vi "transfer char run_subvi_14_2014 05 29_JWa.vi"(0 "VISA session":refnum<visa-resource-name>="GPIB0::17::INSTR", 1 "Y2 axis settings":T5={"Y2 axis on/off"=FALSE, "MINIMUM"=0.0, "MAXIMUM"=1.0, "Variable name"="Ig", "LIN or LOG axis"="LIN"} {"MAXIMUM" format="%.9f"; "MINIMUM" format="%.9f"}, 3 "LKG Path":path, 5 "Var1 sweep settings":T7={"start"=40.0, "stop"=-40.0, "step (linear only)"=-1.0, "sweep spacing (linear: 0)"=0, "sweep mode"=FALSE, "compliance (V)"=100.0, "compliance (A)"=0.001} {"compliance (A)" format="%^.2e"; "compliance (V)" format="%.2f"; "sweep spacing (linear: 0)" items=["linear", "log 10", "log 25", "log 50"]; "step (linear only)" format="%.2f"; "stop" format="%.2f"; "start" format="%.2f"}, 7 "Var2 step settings":T6={"compliance (A)"=0.001, "compliance (V)"=100.0, "start"=-2.0, "total points"=2, "step"=-38.0} {"step" format="%.2f"; "start" format="%.2f"; "compliance (V)" format="%.2f"; "compliance (A)" format="%^.2e"}, 9 "integration time":u32(slide) scale=0.0..2.0, 11 "Input Path":path, 12 "Dielectric Constant":dbl=5.0, 13 "Sample Properties:":T4 {"Date Created" format="%<%x>T"}) -> (2 "Check Cluster":T2, 4 "Output":T3 {"Mobility-Lin" format="%#_4e"; "Mobility-Sat" format="%#_4e"}, 6 "Graph Cluster":T1, 15 "error?":errorcluster)   [LabVIEW 2012]
uses:
  <vilib>/Utility/file.llb/Write To Spreadsheet File (DBL).vi
panel:
  out "concatenated string":string
  in  "Output Path":path
  in  "Temp (K)":dbl=0.001 format="%^.2e"
  in  "NumPts":dbl=5.0
  out "Numeric":dbl
  out "min r":dbl
  out "max r":dbl
  out "error? 2":errorcluster
  in  "MAXIMUM":ext format="%.2e"
  in  "MINIMUM":ext=-1e-05 format="%_2e"
  out "Gate Current Plot":cluster{"trace":dbl[], "trace":dbl[]}(graph)
  in  "Y1 axis":string="Id"
  out "graphic display":cluster{"trace":dbl[], "trace":dbl[]}(graph)
  in  "wait time parameter":dbl=1.0
  in  "Value (Either V or A) 4":dbl
  in  "Value (Either V or A) 3":dbl
  in  "Value (Either V or A) 2":dbl
  in  "Value (V or A)":dbl
  in  "compliance (A)":dbl=0.001 format="%^.2e"
  in  "compliance (V)":dbl=100.0 format="%^.2e"
  in  "Iname":string="Is"
  in  "Vname":string="Vs"
  in  "Function":u16(ring)=4 items=["disabled", "Var1", "Var2", "Var1'", "Constant"]
  in  "Mode":u16(ring)=4 items=["V", "I", "VPulse", "IPulse", "Common"]
  in  "Iname 4":string="I4"
  in  "Vname 4":string="V4"
  in  "Function 4":u16(ring)=4 items=["disabled", "Var1", "Var2", "Var1'", "Constant"]
  in  "Mode 4":u16(ring) items=["V", "I", "VPulse", "IPulse", "Common"]
  in  "Iname 3":string="Ig"
  in  "Vname 3":string="Vg"
  in  "Function 3":u16(ring)=1 items=["disabled", "Var1", "Var2", "Var1'", "Constant"]
  in  "Mode 3":u16(ring) items=["V", "I", "VPulse", "IPulse", "Common"]
  in  "Iname 2":string="Id"
  in  "Vname 2":string="Vd"
  in  "Function 2":u16(ring)=2 items=["disabled", "Var1", "Var2", "Var1'", "Constant"]
  in  "Mode 2":u16(ring) items=["V", "I", "VPulse", "IPulse", "Common"]
  in  "reset":bool=TRUE
  # "SMU1"
  # "SMU2"
  # "SMU3"
  # "SMU4"
  # "Sample Properties:"
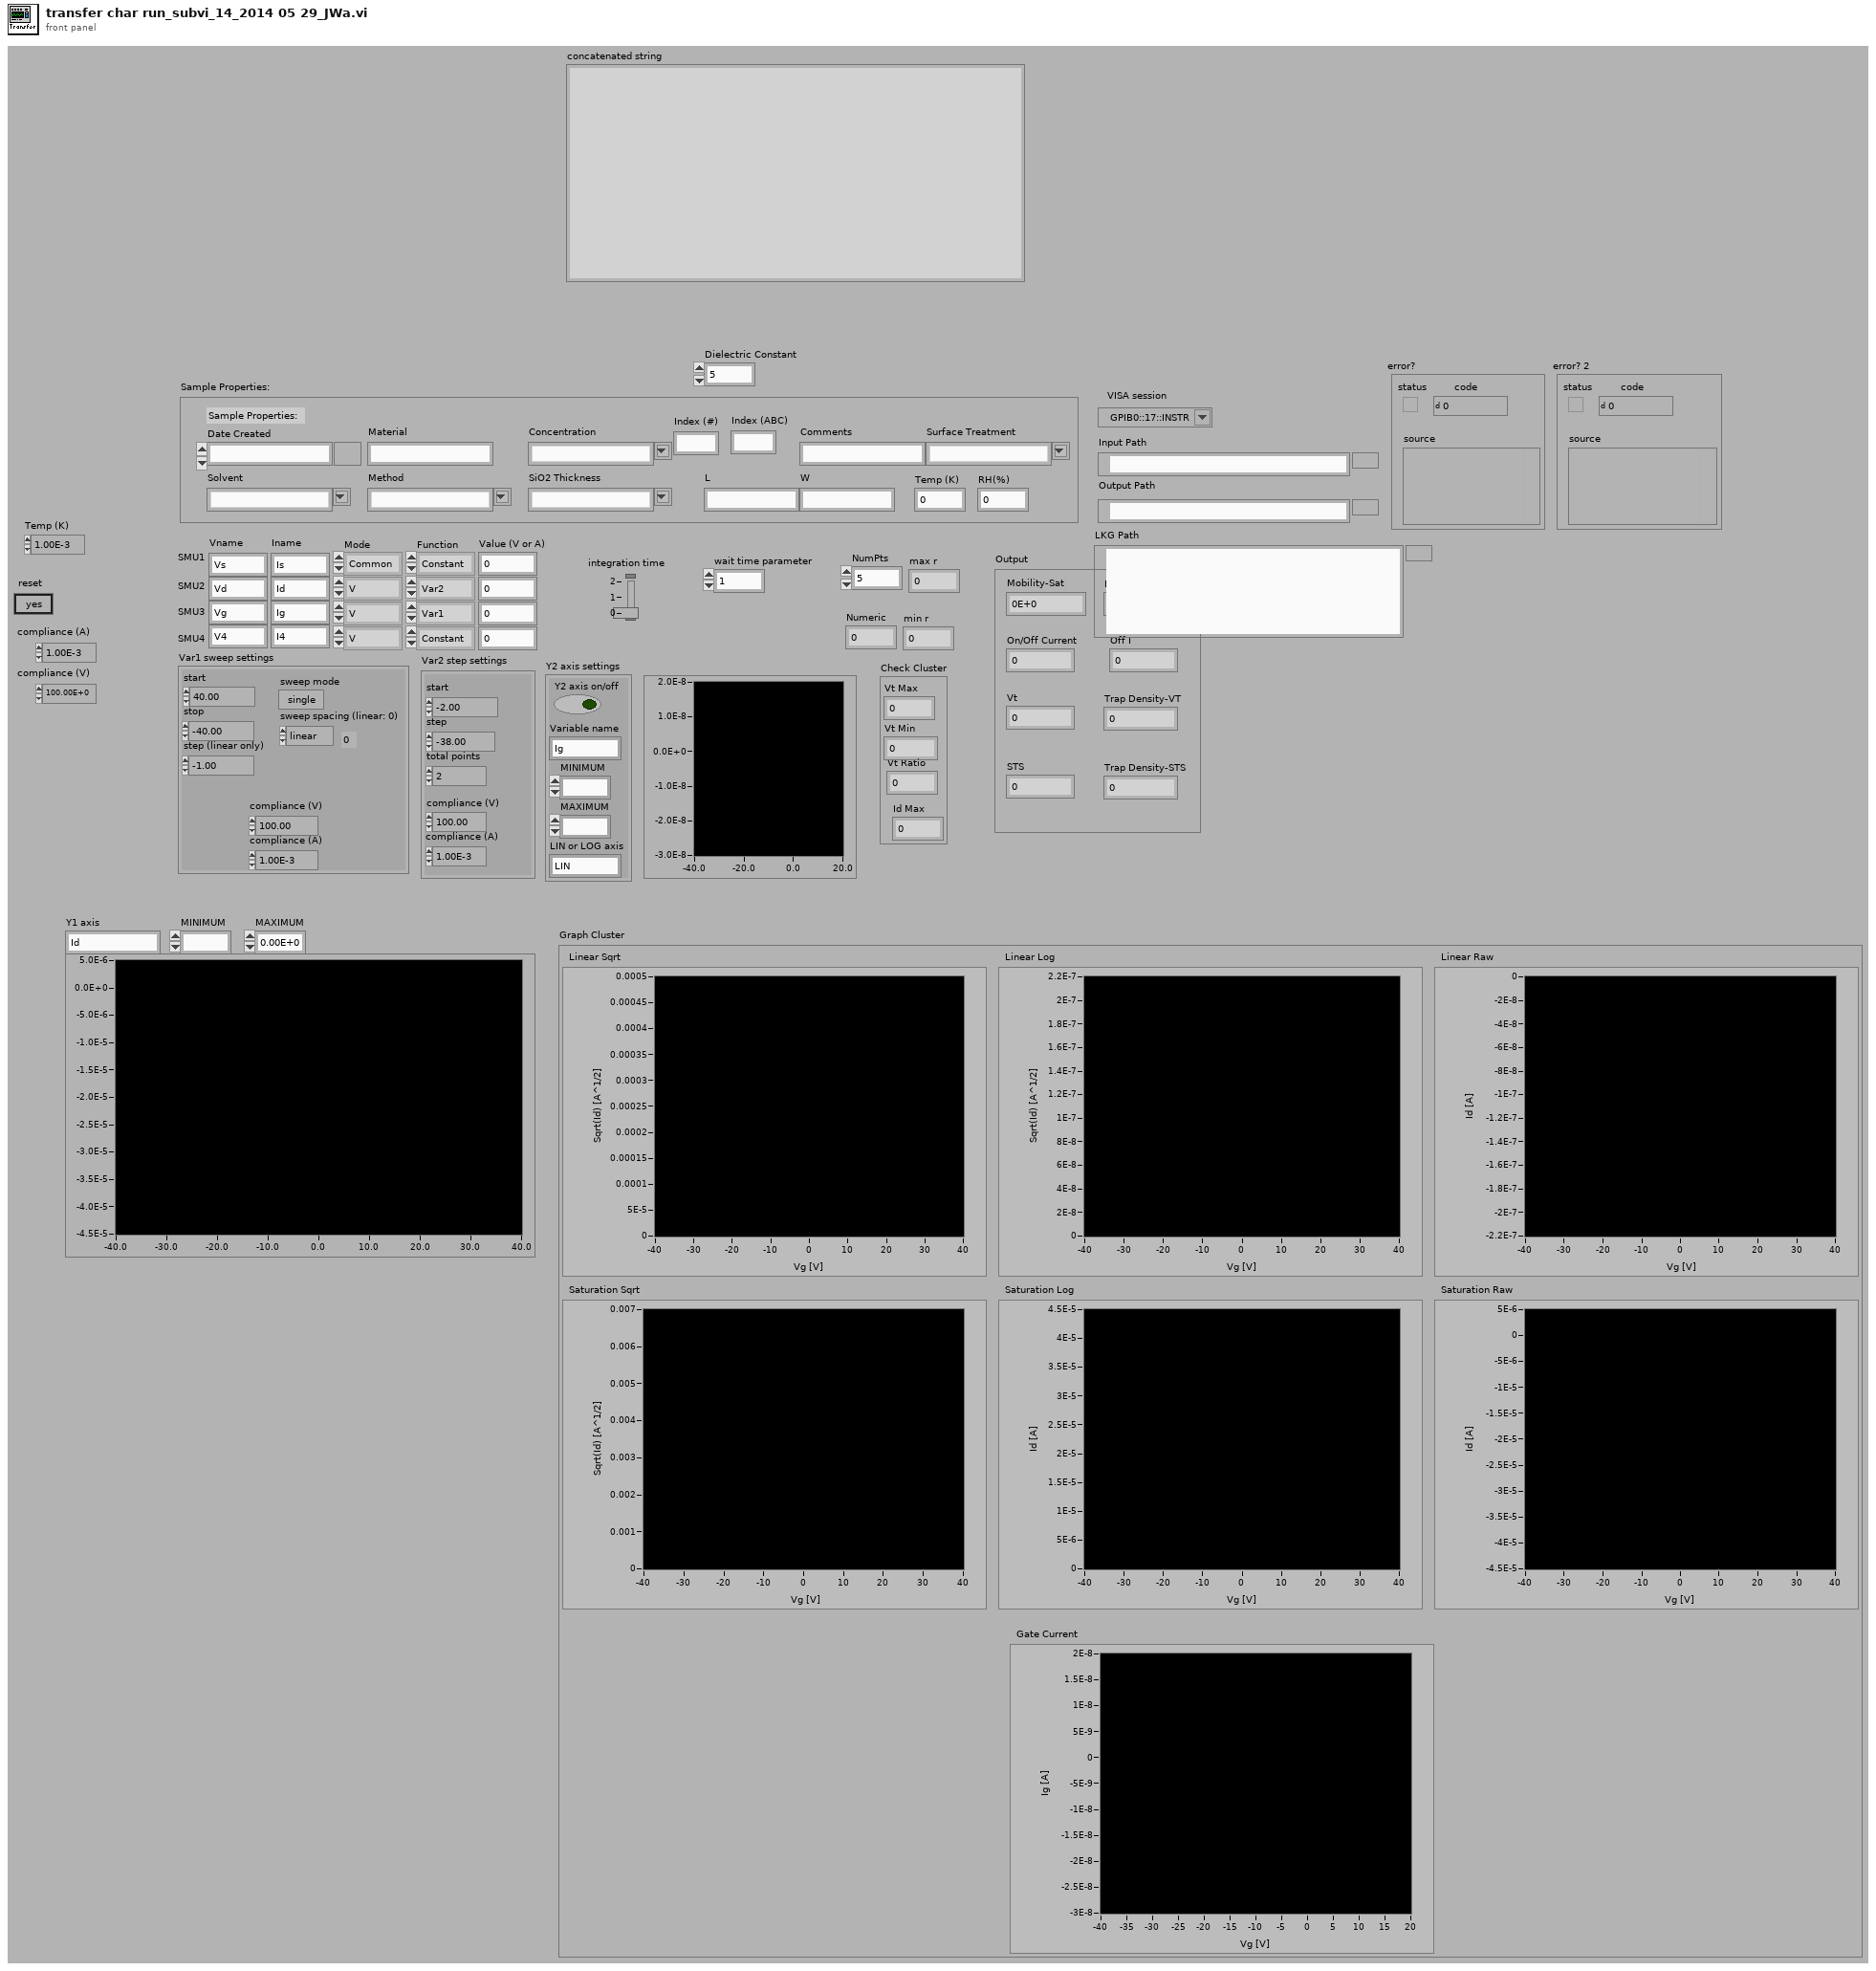
[diagram p1: front panel]
types:
  T1 = cluster{"Linear Sqrt":cluster{dbl[], "trace":dbl[]}[], "Linear Log":cluster{dbl[], "trace":dbl[]}[], "Linear Raw":cluster{dbl[], dbl[]}[], "Saturation Sqrt":cluster{dbl[], "trace":dbl[]}[], "Saturation Log":cluster{dbl[], "trace":dbl[]}[], "Saturation Raw":cluster{dbl[], "trace":dbl[]}[], "Gate Current":cluster{dbl[], "trace":dbl[]}[]}
  T2 = cluster{"Vt Max":i32, "Vt Min":i32, "Vt Ratio":i32, "Id Max":dbl}
  T3 = cluster{"Mobility-Sat":dbl, "Mobility-Lin":dbl, "On/Off Current":dbl, "Off I":dbl, "Vt":dbl, "STS":dbl, "Trap Density-VT":dbl, "Trap Density-STS":dbl}
  T4 = cluster{"Date Created":timestamp, "Material":string, "Solvent":string, "Concentration":string, "Method":string, "SiO2 Thickness":string, "Index (#)":string, "Index (ABC)":string, "L":string, "W":string, "Surface Treatment":string, "Comments":string, "Temp (K)":dbl, "RH(%)":dbl}
  T5 = cluster{"Y2 axis on/off":bool, "MINIMUM":ext, "MAXIMUM":ext, "Variable name":string, "LIN or LOG axis":string}
  T6 = cluster{"compliance (A)":dbl, "compliance (V)":dbl, "start":dbl, "total points":u16, "step":dbl}
  T7 = cluster{"start":dbl, "stop":dbl, "step (linear only)":dbl, "sweep spacing (linear: 0)":u16, "sweep mode":bool, "compliance (V)":dbl, "compliance (A)":dbl}
  T8 = cluster{"Vt Max":dbl, "Vt Min":dbl, "Vt Ratio":dbl, "Id Max":dbl}
  T9 = cluster{"Mobility-Sat":dbl, "Mobility-Lin":dbl, "On/Off I-Sat":dbl, "Off I-Sat":dbl, "VT-Sat":dbl, "Sub Threshold Swing":dbl, "Trap Density-VT":dbl, "Trap Density (N)":dbl}
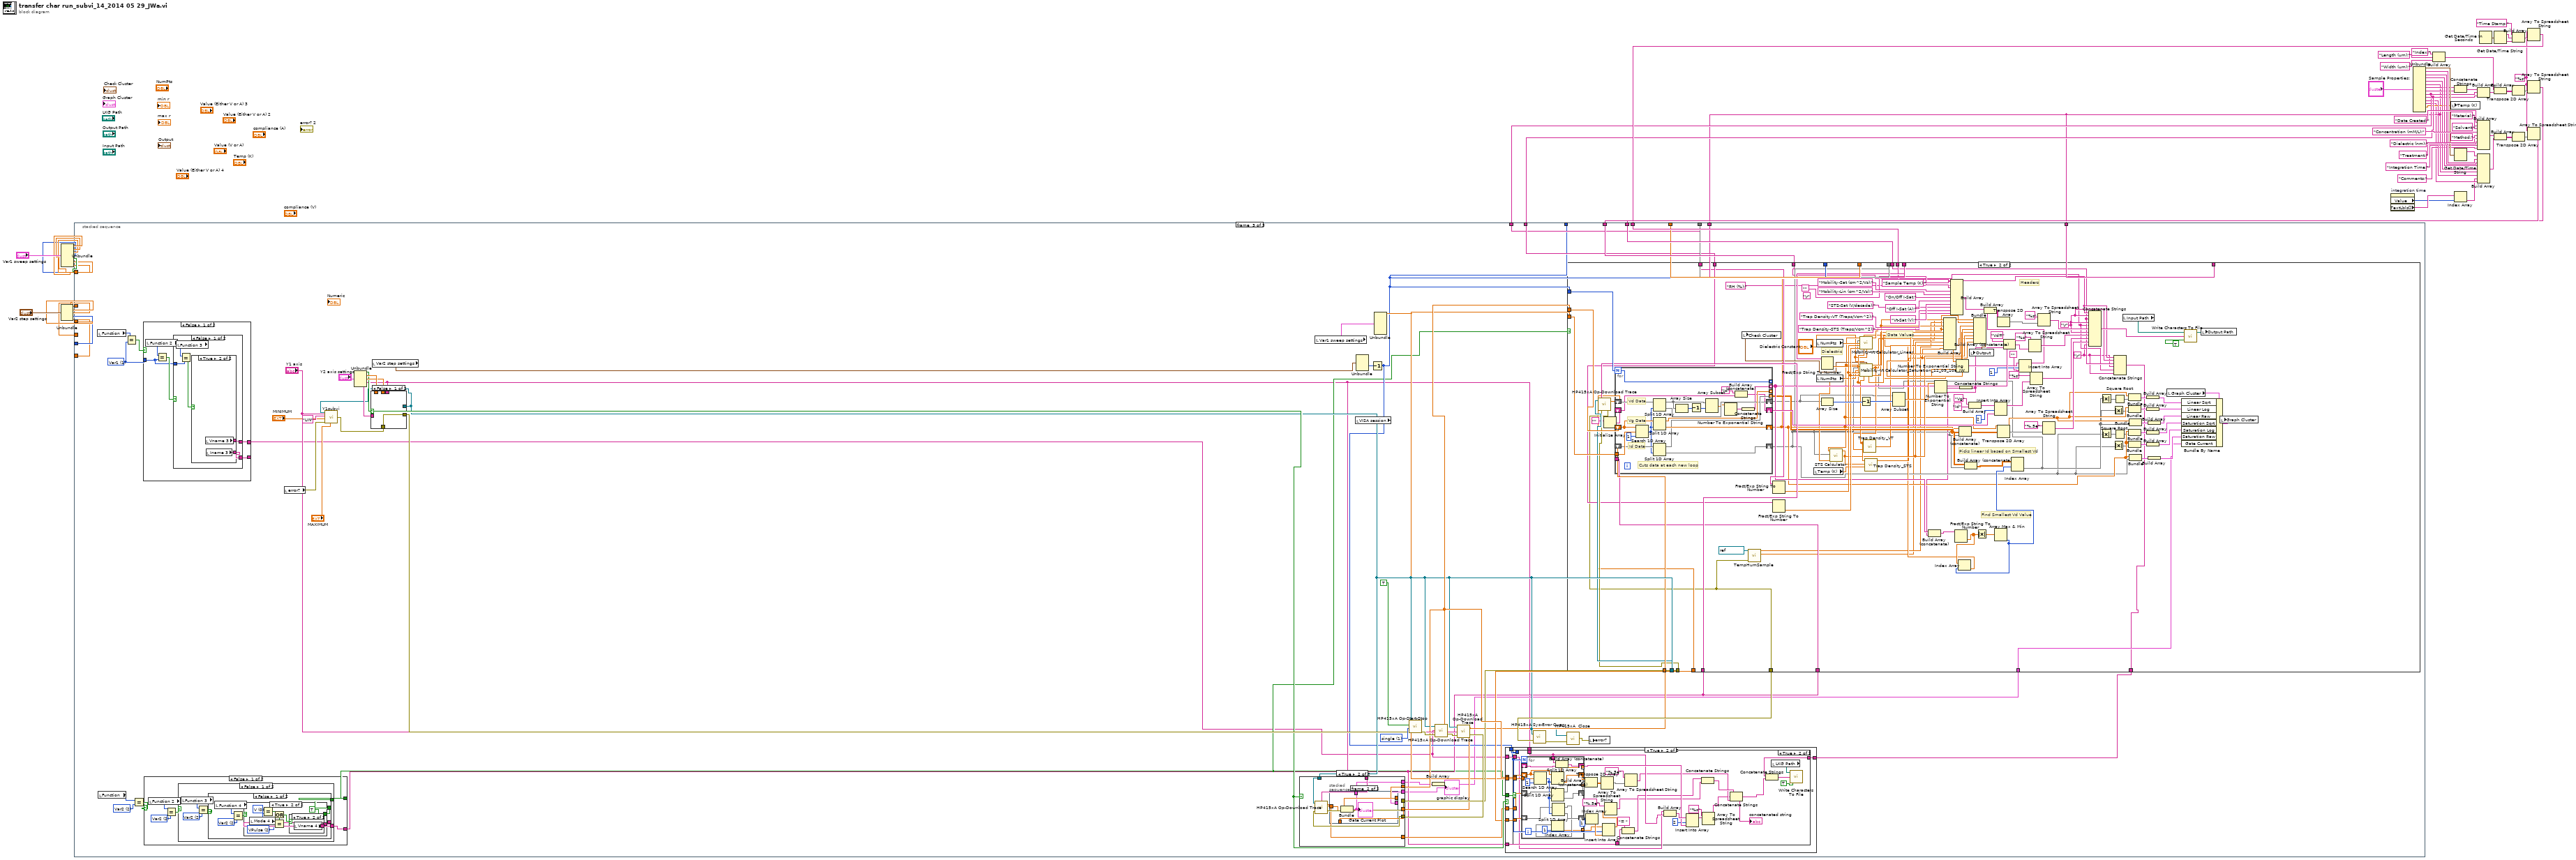
[diagram p0: block diagram]
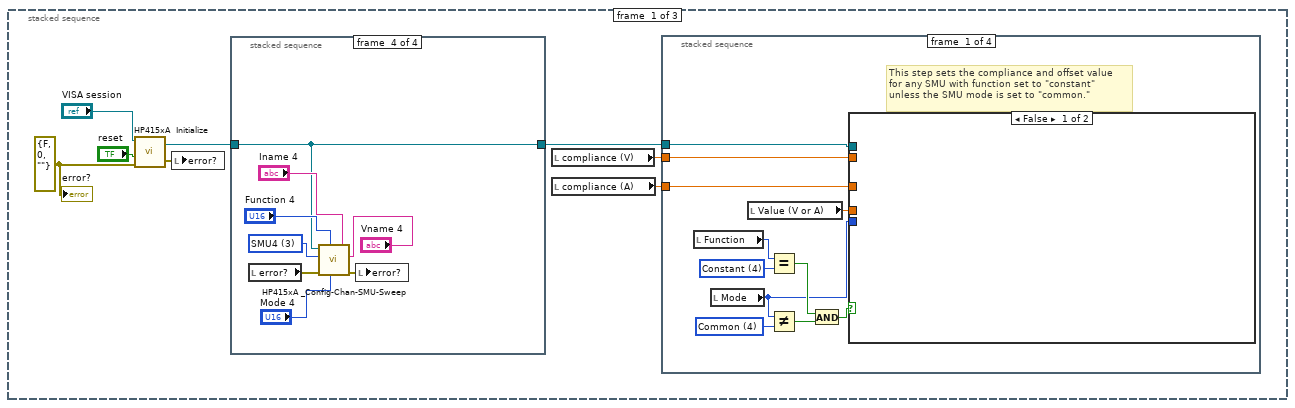
[diagram p2: hidden frame]
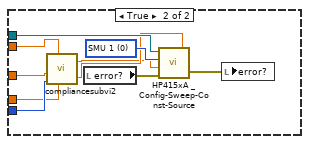
[diagram p3: hidden frame]
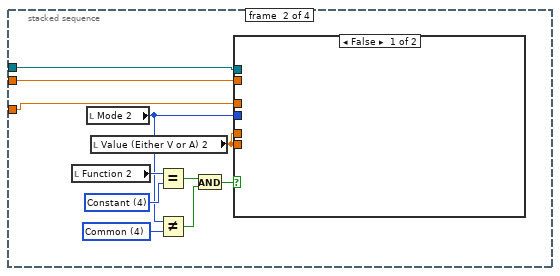
[diagram p4: hidden frame]
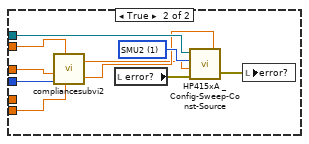
[diagram p5: hidden frame]
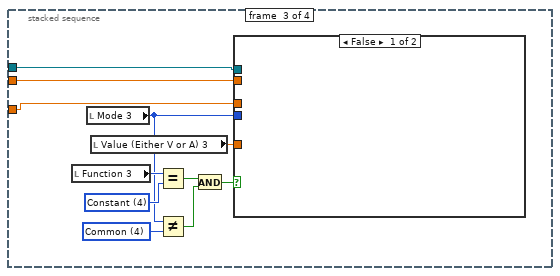
[diagram p6: hidden frame]
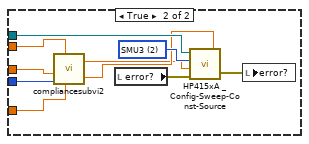
[diagram p7: hidden frame]
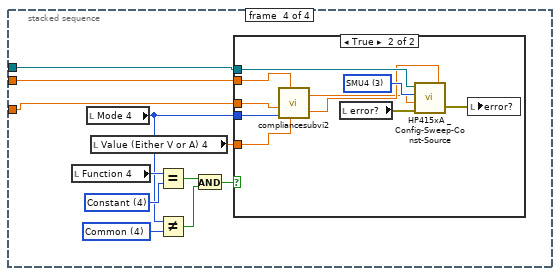
[diagram p8: hidden frame]
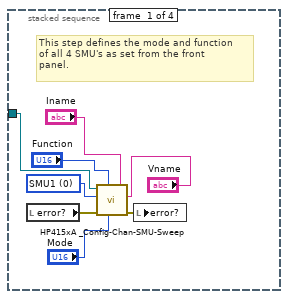
[diagram p10: hidden frame]
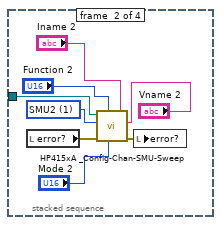
[diagram p11: hidden frame]
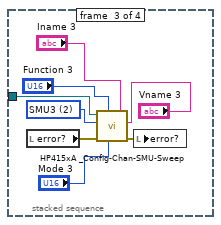
[diagram p12: hidden frame]
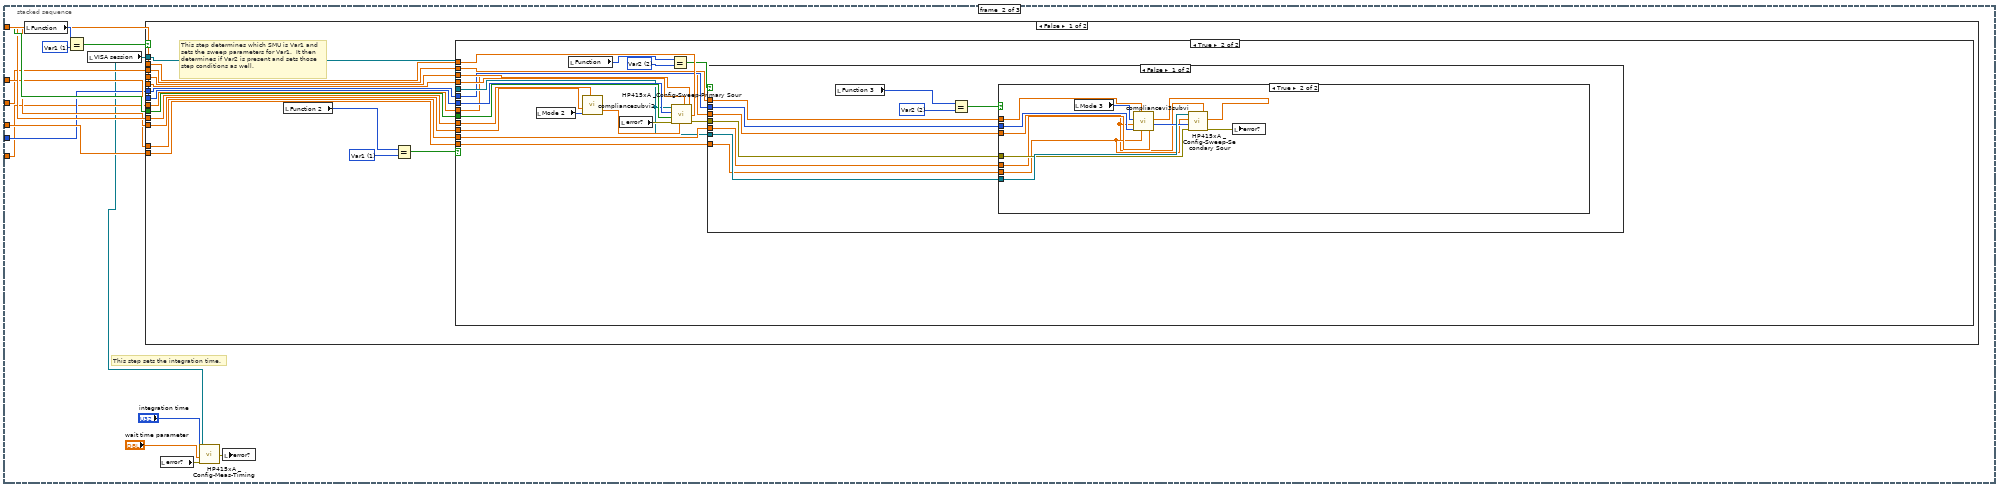
[diagram p13: hidden frame]
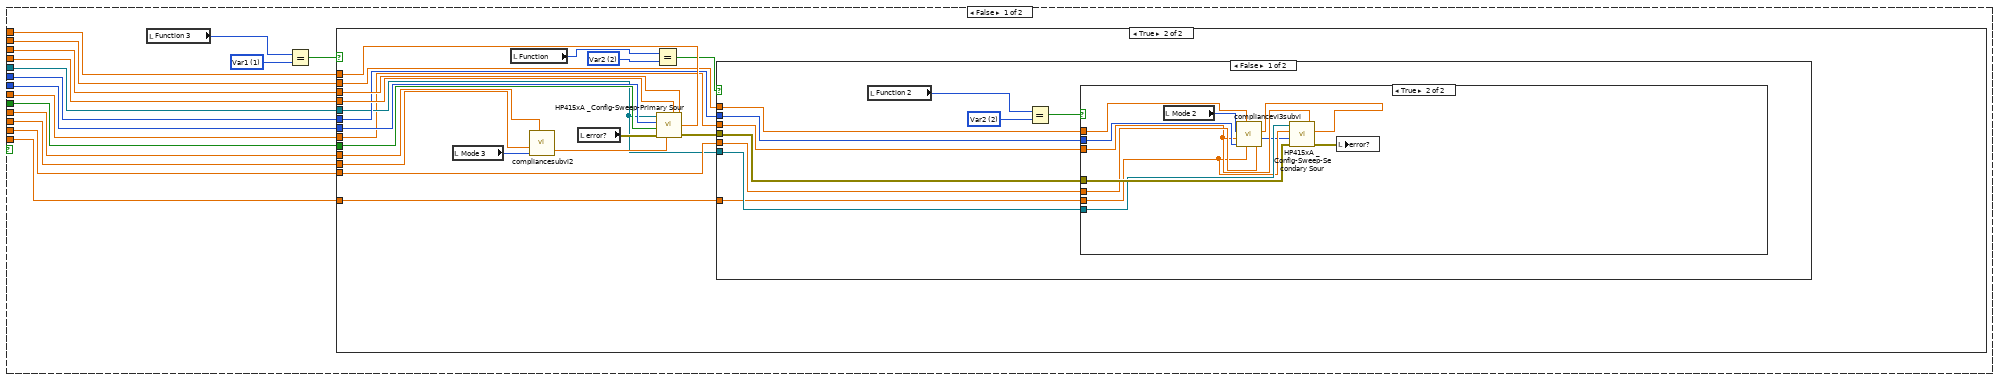
[diagram p14: hidden frame]
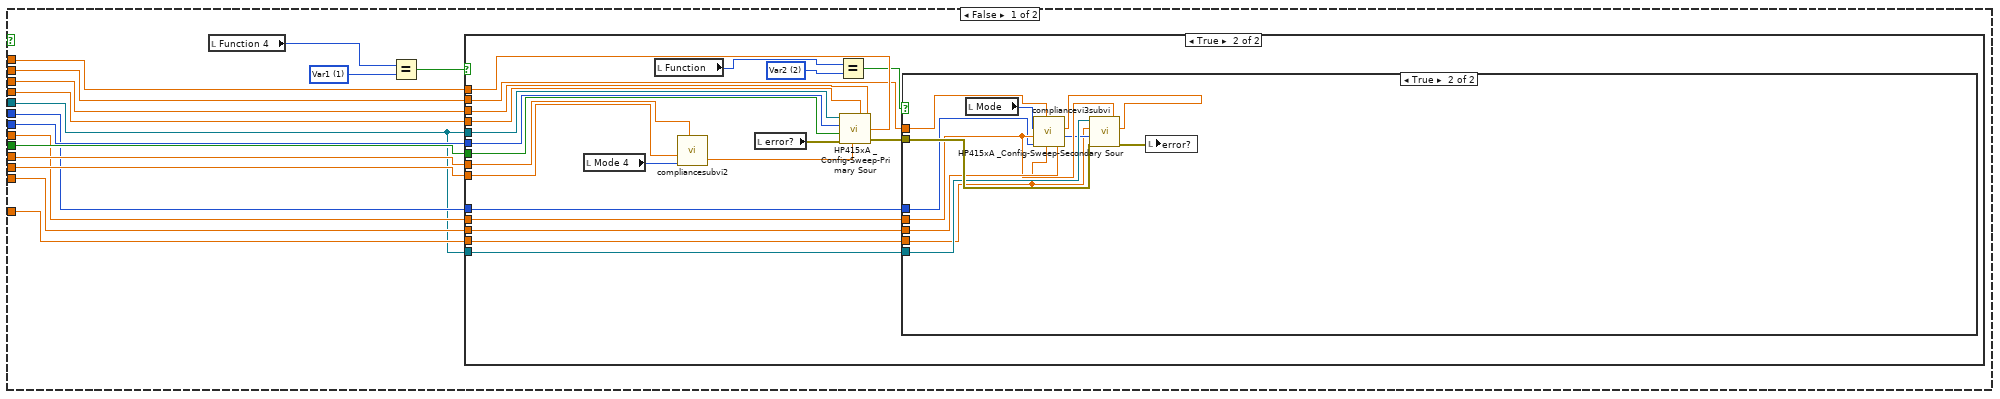
[diagram p15: hidden frame]
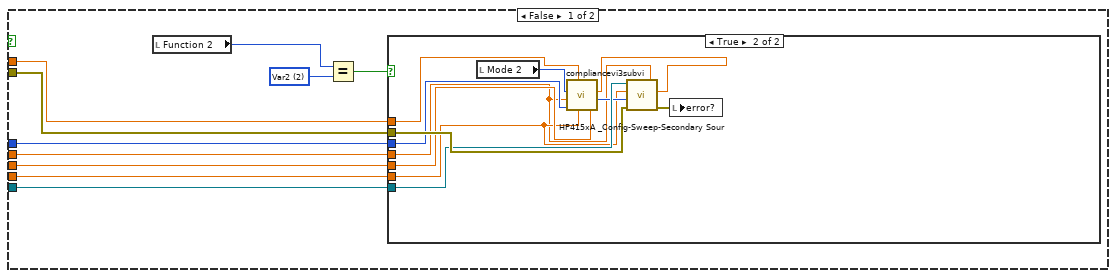
[diagram p17: hidden frame]
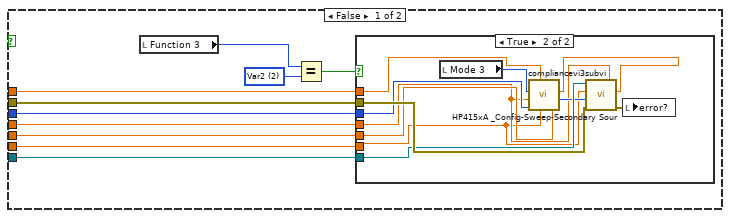
[diagram p18: hidden frame]
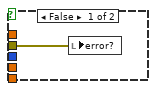
[diagram p19: hidden frame]
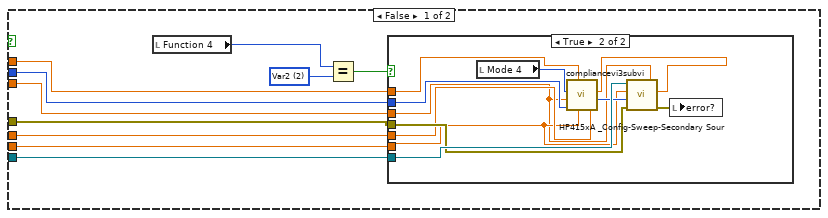
[diagram p20: hidden frame]
diagram:
  w7 = "%s"
  n1 = Unbundle("Var2 step settings") -> ("compliance (A)"=w53:dbl, "compliance (V)"=w52:dbl, "start"=w51:dbl, "total points"=w50:u16, "step"=w49:dbl)
  n2 = Unbundle("Var1 sweep settings") -> ("start"=w61:dbl, "stop"=w60:dbl, "step (linear only)"=w59:dbl, "sweep spacing (linear: 0)"=w58:u16, "sweep mode"=w57:bool, "compliance (V)"=w56:dbl, "compliance (A)"=w55:dbl)
  n3 = property on="integration time" class="Slide (strict)"() -> ("Value"=w2:u32, "TextLbls[]"=w3:string[])  [unwired: 2 in, 2 out]
  n4 = Unbundle("Sample Properties:") -> ("Date Created"=w21:timestamp, "Material"=w20:string, "Solvent"=w17:string, "Concentration"=w16:string, "Method"=w19:string, "SiO2 Thickness"=w8:string, "Index (#)"=w12:string, "Index (ABC)"=w11:string, "L"=w14:string, "W"=w15:string, "Surface Treatment"=w13:string, "Comments"=w4:string, "Temp (K)"=w9:dbl)  [unwired: 1 out]
  n5 = Build Array("Index:", "Length (um):", "Width (um):") -> (w27:string[])
  n6 = local write "Temp (K)"(w9) -> ()
  n7 = Concatenate Strings(w12, w11) -> (w10:string)
  n8 = Index Array(array=w3, index=w2) -> (element=w1:string)
  n9 = Get Date/Time String(seconds (now)=w21) -> (date string=w47:string)  [unwired: 2 in, 1 out]
  n10 = Build Array("Date Created:", "Material:", "Solvent:", "Concentration (mM/L):", "Method:", "Dielectric (nm):", "Treatment:", "Integration Time:", "Comments:") -> (w31:string[])
  n11 = Build Array(w47, w20, w17, w16, w19, w8, w13, w1, w4) -> (w30:string[])
  n12 = Build Array(w10, w14, w15) -> (w26:string[])
  n13 = Get Date/Time In Seconds() -> (seconds since 1Jan1904=w42:timestamp)
  n14 = Get Date/Time String(seconds (now)=w42) -> (date string=w41:string, time string=w40:string)  [unwired: 2 in]
  n15 = Build Array(w27, w26) -> (w25:string[][])
  n16 = Build Array(w31, w30) -> (w29:string[][])
  n17 = Build Array("Time Stamp:", w41, w40) -> (w39:string[])
  n18 = Transpose 2D Array(2D array=w25) -> (transposed array=w24:string[][])
  n19 = Transpose 2D Array(2D array=w29) -> (transposed array=w28:string[][])
  n20 = Array To Spreadsheet String(array=w39, 3:w7) -> (spreadsheet string=w32:string)  [unwired: 1 in]
  n21 = Array To Spreadsheet String(array=w24, 3:w7) -> (spreadsheet string=w23:string)  [unwired: 1 in]
  n22 = Array To Spreadsheet String(array=w28, 3:w7) -> (spreadsheet string=w35:string)  [unwired: 1 in]
  n23 = stacked-sequence {
    tunnel: w61 -> [_ w203 _]
    tunnel: w60 -> [_ w202 _]
    tunnel: w59 -> [_ w201 _]
    tunnel: w58 -> [_ w200 _]
    tunnel: w57 -> [_ w199 _]
    tunnel: w56 -> [_ w198 _]
    tunnel: w55 -> [_ w197 _]
    tunnel: w53 -> [_ w196 _]
    tunnel: w52 -> [_ w195 _]
    tunnel: w51 -> [_ w194 _]
    tunnel: w50 -> [_ w193 _]
    tunnel: w49 -> [_ w192 _]
    tunnel: w32 -> [_ _ w569]
    tunnel: w35 -> [_ _ w568]
    tunnel: w23 -> [_ _ w567]
    tunnel: [_ _ w566] -> _
    tunnel: [_ _ w565] -> _
    tunnel: [_ _ w562] -> _
    tunnel: w15 -> [_ _ w564]
    tunnel: w14 -> [_ _ w563]
    tunnel: w8 -> [_ _ w561]
    tunnel: w8 -> [_ _ w560]
    frame #0 {
      w69 = errorcluster {"status"=FALSE, "code"=0, "source"=""} ("error out")
      n24 = call "HP415xA  Initialize.vi"("instrument descriptor"="VISA session", "reset"="reset", "error in (no error)"=w69) -> ("VISA session"=w66:refnum<visa-resource-name>, "error out"=w68:errorcluster)  [unwired: 2 in]
      n25 = local write "error?"(w68) -> ()
      n26 = stacked-sequence {
        tunnel: w66 -> [w155 w163 w171 w179]
        tunnel: [_ _ _ w179] -> w63
        frame #0 {
          w162 = u32 0 items=["SMU1  ", "SMU2  ", "SMU3  ", "SMU4  ", "SMU5  ", "SMU6  "] ("unit to configure")
          # "This step defines the mode and function\nof all 4 SMU's as set from the front\npanel."
          n27 = local read "error?"() -> (w157:errorcluster)
          n28 = call "HP415xA _Config-Chan-SMU-Sweep.vi"("V name (max 6 chars)"="Vname", "I name (max 6 chars)"="Iname", "mode"="Mode", "function"="Function", "error in (no error)"=w157, "unit to configure"=w162, "VISA session"=w155) -> ("error out"=w156:errorcluster)  [unwired: 2 in]
          n29 = local write "error?"(w156) -> ()
        }
        frame #1 {
          w166 = u32 1 items=["SMU1  ", "SMU2  ", "SMU3  ", "SMU4  ", "SMU5  ", "SMU6  "] ("unit to configure")
          n30 = local read "error?"() -> (w164:errorcluster)
          n31 = call "HP415xA _Config-Chan-SMU-Sweep.vi"("V name (max 6 chars)"="Vname 2", "I name (max 6 chars)"="Iname 2", "mode"="Mode 2", "function"="Function 2", "error in (no error)"=w164, "unit to configure"=w166, "VISA session"=w163) -> ("error out"=w165:errorcluster)  [unwired: 2 in]
          n32 = local write "error?"(w165) -> ()
        }
        frame #2 {
          w174 = u32 2 items=["SMU1  ", "SMU2  ", "SMU3  ", "SMU4  ", "SMU5  ", "SMU6  "] ("unit to configure")
          n33 = local read "error?"() -> (w172:errorcluster)
          n34 = call "HP415xA _Config-Chan-SMU-Sweep.vi"("V name (max 6 chars)"="Vname 3", "I name (max 6 chars)"="Iname 3", "mode"="Mode 3", "function"="Function 3", "error in (no error)"=w172, "unit to configure"=w174, "VISA session"=w171) -> ("error out"=w173:errorcluster)  [unwired: 2 in]
          n35 = local write "error?"(w173) -> ()
        }
        frame #3 {
          w182 = u32 3 items=["SMU1  ", "SMU2  ", "SMU3  ", "SMU4  ", "SMU5  ", "SMU6  "] ("unit to configure")
          n36 = local read "error?"() -> (w181:errorcluster)
          n37 = call "HP415xA _Config-Chan-SMU-Sweep.vi"("V name (max 6 chars)"="Vname 4", "I name (max 6 chars)"="Iname 4", "mode"="Mode 4", "function"="Function 4", "error in (no error)"=w181, "unit to configure"=w182, "VISA session"=w179) -> ("error out"=w180:errorcluster)  [unwired: 2 in]
          n38 = local write "error?"(w180) -> ()
        }
      }
      n39 = local read "compliance (V)"() -> (w65:dbl)
      n40 = local read "compliance (A)"() -> (w64:dbl)
      n41 = stacked-sequence {
        tunnel: w63 -> [w79 w99 w118 w138]
        tunnel: w64 -> [w73 w95 w116 w136]
        tunnel: w65 -> [w72 w94 w115 w137]
        frame #0 {
          w77 = u16 4 items=["V", "I", "VPulse", "IPulse", "Common"] ("Mode")
          w81 = u16 4 items=["disabled", "Var1", "Var2", "Var1'", "Constant"] ("Function")
          # "This step sets the compliance and offset value\nfor any SMU with function set to \"constant\"\nunless the SMU mode is set to \"common.\""
          n42 = local read "Function"() -> (w80:u16)
          n43 = local read "Mode"() -> (w71:u16)
          n44 = local read "Value (V or A)"() -> (w74:dbl)
          n45 = Equal?(x=w80, y=w81) -> (x = y?=w78:bool)
          n46 = Not Equal?(x=w71, y=w77) -> (x != y?=w76:bool)
          n47 = And(x=w78, y=w76) -> (x .and. y?=w75:bool)
          n48 = case shown="False" w75 {
            tunnel: w79 -> [_ w91]
            tunnel: w72 -> [_ w87]
            tunnel: w73 -> [_ w86]
            tunnel: w74 -> [_ w83]
            tunnel: w71 -> [_ w84]
            frame False {
            }
            frame True {
              w90 = u16 0 items=["SMU 1", "SMU2", "SMU3", "SMU4", "SMU5", "SMU6", "VSU1", "VSU2"] ("unit (SMU1:0)")
              n49 = call "compliancesubvi2.vi"("Value1"=w83, "compliance (V)"=w87, "Mode"=w84, "compliance (A)"=w86) -> ("compliance"=w85:dbl, "constant"=w82:dbl)  [unwired: 2 in]
              n50 = local read "error?"() -> (w89:errorcluster)
              n51 = call "HP415xA _Config-Sweep-Const-Source.vi"("compliance (SMUs only)"=w85, "error in (no error)"=w89, "source (V or A)"=w82, "unit (SMU1:0)"=w90, "VISA session"=w91) -> ("error out"=w88:errorcluster)
              n52 = local write "error?"(w88) -> ()
            }
          }
        }
        frame #1 {
          w96 = u16 4 items=["V", "I", "VPulse", "IPulse", "Common"] ("Mode 2")
          w97 = u16 4 items=["disabled", "Var1", "Var2", "Var1'", "Constant"] ("Function 2")
          n53 = local read "Function 2"() -> (w98:u16)
          n54 = local read "Mode 2"() -> (w93:u16)
          n55 = local read "Value (Either V or A) 2"() -> (w92:dbl)
          n56 = Equal?(x=w98, y=w97) -> (x = y?=w102:bool)
          n57 = Not Equal?(x=w93, y=w96) -> (x != y?=w101:bool)
          n58 = And(x=w102, y=w101) -> (x .and. y?=w100:bool)
          n59 = case shown="False" w100 {
            tunnel: w99 -> [_ w112]
            tunnel: w94 -> [_ w110]
            tunnel: w95 -> [_ w109]
            tunnel: w92 -> [_ _]
            tunnel: w93 -> [_ w105]
            tunnel: w92 -> [_ w104]
            frame False {
            }
            frame True {
              w111 = u16 1 items=["SMU 1", "SMU2", "SMU3", "SMU4", "SMU5", "SMU6", "VSU1", "VSU2"] ("unit (SMU1:0)")
              n60 = call "compliancesubvi2.vi"("Value1"=w104, "compliance (V)"=w110, "Mode"=w105, "compliance (A)"=w109) -> ("compliance"=w108:dbl, "constant"=w103:dbl)  [unwired: 2 in]
              n61 = local read "error?"() -> (w107:errorcluster)
              n62 = call "HP415xA _Config-Sweep-Const-Source.vi"("compliance (SMUs only)"=w108, "error in (no error)"=w107, "source (V or A)"=w103, "unit (SMU1:0)"=w111, "VISA session"=w112) -> ("error out"=w106:errorcluster)
              n63 = local write "error?"(w106) -> ()
            }
          }
        }
        frame #2 {
          w120 = u16 4 items=["V", "I", "VPulse", "IPulse", "Common"] ("Mode 2")
          w121 = u16 4 items=["disabled", "Var1", "Var2", "Var1'", "Constant"] ("Function 2")
          n64 = local read "Function 3"() -> (w119:u16)
          n65 = local read "Mode 3"() -> (w114:u16)
          n66 = local read "Value (Either V or A) 3"() -> (w117:dbl)
          n67 = Equal?(x=w119, y=w121) -> (x = y?=w123:bool)
          n68 = Not Equal?(x=w114, y=w120) -> (x != y?=w122:bool)
          n69 = And(x=w123, y=w122) -> (x .and. y?=w113:bool)
          n70 = case shown="False" w113 {
            tunnel: w118 -> [_ w131]
            tunnel: w117 -> [_ w125]
            tunnel: w116 -> [_ w128]
            tunnel: w115 -> [_ w127]
            tunnel: w114 -> [_ w126]
            frame False {
            }
            frame True {
              w130 = u16 2 items=["SMU 1", "SMU2", "SMU3", "SMU4", "SMU5", "SMU6", "VSU1", "VSU2"] ("unit (SMU1:0)")
              n71 = call "compliancesubvi2.vi"("Value1"=w125, "compliance (V)"=w127, "Mode"=w126, "compliance (A)"=w128) -> ("compliance"=w129:dbl, "constant"=w124:dbl)  [unwired: 2 in]
              n72 = local read "error?"() -> (w133:errorcluster)
              n73 = call "HP415xA _Config-Sweep-Const-Source.vi"("compliance (SMUs only)"=w129, "error in (no error)"=w133, "source (V or A)"=w124, "unit (SMU1:0)"=w130, "VISA session"=w131) -> ("error out"=w132:errorcluster)
              n74 = local write "error?"(w132) -> ()
            }
          }
        }
        frame #3 {
          w140 = u16 4 items=["V", "I", "VPulse", "IPulse", "Common"] ("Mode 4")
          w141 = u16 4 items=["disabled", "Var1", "Var2", "Var1'", "Constant"] ("Function 4")
          n75 = local read "Function 4"() -> (w142:u16)
          n76 = local read "Mode 4"() -> (w135:u16)
          n77 = local read "Value (Either V or A) 4"() -> (w134:dbl)
          n78 = Equal?(x=w142, y=w141) -> (x = y?=w144:bool)
          n79 = Not Equal?(x=w135, y=w140) -> (x != y?=w143:bool)
          n80 = And(x=w144, y=w143) -> (x .and. y?=w139:bool)
          n81 = case shown="True" w139 {
            tunnel: w138 -> [_ w153]
            tunnel: w137 -> [_ w149]
            tunnel: w136 -> [_ w150]
            tunnel: w135 -> [_ w148]
            tunnel: w134 -> [_ w147]
            frame False {
            }
            frame True {
              w154 = u16 3 items=["SMU 1", "SMU2", "SMU3", "SMU4", "SMU5", "SMU6", "VSU1", "VSU2"] ("unit (SMU1:0)")
              n82 = call "compliancesubvi2.vi"("Value1"=w147, "compliance (V)"=w149, "Mode"=w148, "compliance (A)"=w150) -> ("compliance"=w146:dbl, "constant"=w145:dbl)  [unwired: 2 in]
              n83 = local read "error?"() -> (w152:errorcluster)
              n84 = call "HP415xA _Config-Sweep-Const-Source.vi"("compliance (SMUs only)"=w146, "error in (no error)"=w152, "source (V or A)"=w145, "unit (SMU1:0)"=w154, "VISA session"=w153) -> ("error out"=w151:errorcluster)
              n85 = local write "error?"(w151) -> ()
            }
          }
        }
      }
      "error?" <- w69
    }
    frame #1 {
      w206 = u16 1 items=["disabled", "Var1", "Var2", "Var1'", "Constant"] ("Function")
      # "This step sets the integration time."
      n86 = local read "Function"() -> (w205:u16)
      n87 = Equal?(x=w205, y=w206) -> (x = y?=w204:bool)
      n88 = local read "VISA session"() -> (w187:refnum<visa-resource-name>)
      n89 = case shown="False" w204 {
        tunnel: w198 -> [w219 w495]
        tunnel: w197 -> [w220 w494]
        tunnel: w200 -> [w217 w493]
        tunnel: w199 -> [w218 w492]
        tunnel: w201 -> [w214 w491]
        tunnel: w202 -> [w213 w490]
        tunnel: w203 -> [w215 w489]
        tunnel: w187 -> [w216 w478]
        tunnel: w196 -> [w211 w484]
        tunnel: w195 -> [w210 w483]
        tunnel: w194 -> [w209 w482]
        tunnel: w193 -> [w208 w481]
        tunnel: w192 -> [w207 w480]
        frame False {
          w222 = u16 1 items=["disabled", "Var1", "Var2", "Var1'", "Constant"] ("Function")
          # "This step determines which SMU is Var1 and\nsets the sweep parameters for Var1.  It then\ndetermines if Var2 is present and sets those\nstep conditions as well."
          n90 = local read "Function 2"() -> (w221:u16)
          n91 = Equal?(x=w221, y=w222) -> (x = y?=w212:bool)
          n92 = case shown="True" w212 {
            tunnel: w220 -> [w228 w421]
            tunnel: w219 -> [w229 w420]
            tunnel: w218 -> [w230 w419]
            tunnel: w217 -> [w231 w418]
            tunnel: w216 -> [w235 w407]
            tunnel: w215 -> [w234 w417]
            tunnel: w214 -> [w232 w416]
            tunnel: w213 -> [w233 w415]
            tunnel: w211 -> [w227 w410]
            tunnel: w210 -> [w226 w409]
            tunnel: w209 -> [w224 w408]
            tunnel: w208 -> [w225 w405]
            tunnel: w207 -> [w223 w404]
            frame False {
              w238 = u16 1 items=["disabled", "Var1", "Var2", "Var1'", "Constant"] ("Function")
              n93 = local read "Function 3"() -> (w237:u16)
              n94 = Equal?(x=w237, y=w238) -> (x = y?=w236:bool)
              n95 = case shown="True" w236 {
                tunnel: w235 -> [w239 w332]
                tunnel: w234 -> [w251 w349]
                tunnel: w233 -> [w248 w348]
                tunnel: w232 -> [w247 w347]
                tunnel: w231 -> [w250 w346]
                tunnel: w230 -> [w249 w345]
                tunnel: w229 -> [w246 w344]
                tunnel: w228 -> [w245 w343]
                tunnel: w227 -> [w244 w336]
                tunnel: w226 -> [w243 w335]
                tunnel: w225 -> [w242 w334]
                tunnel: w224 -> [w241 w331]
                tunnel: w223 -> [w240 w330]
                frame False {
                  w254 = u16 1 items=["disabled", "Var1", "Var2", "Var1'", "Constant"] ("Function")
                  n96 = local read "Function 4"() -> (w253:u16)
                  n97 = Equal?(x=w253, y=w254) -> (x = y?=w252:bool)
                  n98 = case shown="True" w252 {
                    tunnel: w251 -> [_ w273]
                    tunnel: w239 -> [_ w272]
                    tunnel: w250 -> [_ w271]
                    tunnel: w249 -> [_ w270]
                    tunnel: w248 -> [_ w269]
                    tunnel: w247 -> [_ w268]
                    tunnel: w246 -> [_ w267]
                    tunnel: w245 -> [_ w266]
                    tunnel: w244 -> [_ w261]
                    tunnel: w243 -> [_ w260]
                    tunnel: w242 -> [_ w259]
                    tunnel: w241 -> [_ w258]
                    tunnel: w240 -> [_ w257]
                    tunnel: w239 -> [_ w255]
                    frame False {
                    }
                    frame True {
                      w264 = u16 2 items=["disabled", "Var1", "Var2", "Var1'", "Constant"] ("Function")
                      n99 = local read "Mode 4"() -> (w275:u16)
                      n100 = local read "Function"() -> (w263:u16)
                      n101 = call "compliancesubvi2.vi"("compliance (V)"=w267, "Mode"=w275, "compliance (A)"=w266) -> ("compliance"=w274:dbl)  [unwired: 3 in, 1 out]
                      n102 = local read "error?"() -> (w265:errorcluster)
                      n103 = Equal?(x=w263, y=w264) -> (x = y?=w262:bool)
                      n104 = call "HP415xA _Config-Sweep-Primary Sour.vi"("step (linear only)"=w268, "stop"=w269, "start"=w273, "compliance"=w274, "error in (no error)"=w265, "sweep mode"=w270, "sweep spacing (linear: 0)"=w271, "VISA session"=w272) -> ("error out"=w256:errorcluster)  [unwired: 2 in]
                      n105 = case shown="True" w262 {
                        tunnel: w261 -> [w282 w325]
                        tunnel: w260 -> [w281 w320]
                        tunnel: w259 -> [w280 w319]
                        tunnel: w258 -> [w279 w321]
                        tunnel: w257 -> [w278 w324]
                        tunnel: w256 -> [w277 w327]
                        tunnel: w255 -> [w276 w326]
                        frame False {
                          w285 = u16 2 items=["disabled", "Var1", "Var2", "Var1'", "Constant"] ("Function")
                          n106 = local read "Function 2"() -> (w284:u16)
                          n107 = Equal?(x=w284, y=w285) -> (x = y?=w283:bool)
                          n108 = case shown="True" w283 {
                            tunnel: w282 -> [w293 w313]
                            tunnel: w281 -> [w292 w314]
                            tunnel: w280 -> [w291 w312]
                            tunnel: w279 -> [w290 w310]
                            tunnel: w278 -> [w289 w308]
                            tunnel: w277 -> [w288 w318]
                            tunnel: w276 -> [w286 w317]
                            frame False {
                              w295 = u16 2 items=["disabled", "Var1", "Var2", "Var1'", "Constant"] ("Function")
                              n109 = local read "Function 3"() -> (w287:u16)
                              n110 = Equal?(x=w287, y=w295) -> (x = y?=w294:bool)
                              n111 = case shown="True" w294 {
                                tunnel: w293 -> [_ w301]
                                tunnel: w292 -> [_ w302]
                                tunnel: w291 -> [_ w303]
                                tunnel: w290 -> [_ w297]
                                tunnel: w289 -> [_ w298]
                                tunnel: w288 -> [w296 w307]
                                tunnel: w286 -> [_ w306]
                                frame False {
                                n112 = local write "error?"(w296) -> ()
                                }
                                frame True {
                                n113 = local read "Mode 3"() -> (w305:u16)
                                n114 = call "compliancevi3subvi.vi"("compliance (A)"=w301, "start"=w297, "compliance (V)"=w302, "total points"=w303, "step"=w298, "Mode"=w305) -> ("total points 2"=w300:u16, "compliance"=w299:dbl)  [unwired: 1 in, 1 out]
                                n115 = call "HP415xA _Config-Sweep-Secondary Sour.vi"("compliance"=w299, "step"=w298, "error in (no error)"=w307, "total points"=w300, "start"=w297, "VISA session"=w306) -> ("error out"=w304:errorcluster)  [unwired: 1 in]
                                n116 = local write "error?"(w304) -> ()
                                }
                              }
                            }
                            frame True {
                              n117 = local read "Mode 2"() -> (w316:u16)
                              n118 = call "compliancevi3subvi.vi"("compliance (A)"=w313, "start"=w310, "compliance (V)"=w314, "total points"=w312, "step"=w308, "Mode"=w316) -> ("total points 2"=w311:u16, "compliance"=w309:dbl)  [unwired: 1 in, 1 out]
                              n119 = call "HP415xA _Config-Sweep-Secondary Sour.vi"("compliance"=w309, "step"=w308, "error in (no error)"=w318, "total points"=w311, "start"=w310, "VISA session"=w317) -> ("error out"=w315:errorcluster)  [unwired: 1 in]
                              n120 = local write "error?"(w315) -> ()
                            }
                          }
                        }
                        frame True {
                          n121 = local read "Mode"() -> (w329:u16)
                          n122 = call "compliancevi3subvi.vi"("compliance (A)"=w325, "start"=w321, "compliance (V)"=w320, "total points"=w319, "step"=w324, "Mode"=w329) -> ("total points 2"=w322:u16, "compliance"=w323:dbl)  [unwired: 1 in, 1 out]
                          n123 = call "HP415xA _Config-Sweep-Secondary Sour.vi"("compliance"=w323, "step"=w324, "error in (no error)"=w327, "total points"=w322, "start"=w321, "VISA session"=w326) -> ("error out"=w328:errorcluster)  [unwired: 1 in]
                          n124 = local write "error?"(w328) -> ()
                        }
                      }
                    }
                  }
                }
                frame True {
                  w339 = u16 2 items=["disabled", "Var1", "Var2", "Var1'", "Constant"] ("Function")
                  n125 = local read "Mode 3"() -> (w341:u16)
                  n126 = local read "Function"() -> (w338:u16)
                  n127 = call "compliancesubvi2.vi"("compliance (V)"=w344, "Mode"=w341, "compliance (A)"=w343) -> ("compliance"=w342:dbl)  [unwired: 3 in, 1 out]
                  n128 = local read "error?"() -> (w340:errorcluster)
                  n129 = Equal?(x=w338, y=w339) -> (x = y?=w337:bool)
                  n130 = call "HP415xA _Config-Sweep-Primary Sour.vi"("step (linear only)"=w347, "stop"=w348, "start"=w349, "compliance"=w342, "error in (no error)"=w340, "sweep mode"=w345, "sweep spacing (linear: 0)"=w346, "VISA session"=w332) -> ("error out"=w333:errorcluster)  [unwired: 2 in]
                  n131 = case shown="False" w337 {
                    tunnel: w336 -> [w354 w399]
                    tunnel: w335 -> [w353 w398]
                    tunnel: w334 -> [w351 w397]
                    tunnel: w333 -> [w356 w402]
                    tunnel: w332 -> [w355 w401]
                    tunnel: w331 -> [w350 w394]
                    tunnel: w330 -> [w352 w393]
                    frame False {
                      w359 = u16 2 items=["disabled", "Var1", "Var2", "Var1'", "Constant"] ("Function")
                      n132 = local read "Function 2"() -> (w358:u16)
                      n133 = Equal?(x=w358, y=w359) -> (x = y?=w357:bool)
                      n134 = case shown="True" w357 {
                        tunnel: w356 -> [w366 w391]
                        tunnel: w355 -> [w365 w390]
                        tunnel: w354 -> [w364 w386]
                        tunnel: w353 -> [w363 w387]
                        tunnel: w352 -> [w360 w385]
                        tunnel: w351 -> [w362 w388]
                        tunnel: w350 -> [w361 w384]
                        frame False {
                          w369 = u16 2 items=["disabled", "Var1", "Var2", "Var1'", "Constant"] ("Function")
                          n135 = local read "Function 4"() -> (w368:u16)
                          n136 = Equal?(x=w368, y=w369) -> (x = y?=w367:bool)
                          n137 = case shown="True" w367 {
                            tunnel: w366 -> [w370 w379]
                            tunnel: w365 -> [_ w380]
                            tunnel: w364 -> [_ w376]
                            tunnel: w363 -> [_ w377]
                            tunnel: w362 -> [_ w375]
                            tunnel: w361 -> [_ w372]
                            tunnel: w360 -> [_ w371]
                            frame False {
                              n138 = local write "error?"(w370) -> ()
                            }
                            frame True {
                              n139 = local read "Mode 4"() -> (w381:u16)
                              n140 = call "compliancevi3subvi.vi"("compliance (A)"=w376, "start"=w372, "compliance (V)"=w377, "total points"=w375, "step"=w371, "Mode"=w381) -> ("total points 2"=w374:u16, "compliance"=w373:dbl)  [unwired: 1 in, 1 out]
                              n141 = call "HP415xA _Config-Sweep-Secondary Sour.vi"("compliance"=w373, "step"=w371, "error in (no error)"=w379, "total points"=w374, "start"=w372, "VISA session"=w380) -> ("error out"=w378:errorcluster)  [unwired: 1 in]
                              n142 = local write "error?"(w378) -> ()
                            }
                          }
                        }
                        frame True {
                          n143 = local read "Mode 2"() -> (w392:u16)
                          n144 = call "compliancevi3subvi.vi"("compliance (A)"=w386, "start"=w384, "compliance (V)"=w387, "total points"=w388, "step"=w385, "Mode"=w392) -> ("total points 2"=w383:u16, "compliance"=w382:dbl)  [unwired: 1 in, 1 out]
                          n145 = call "HP415xA _Config-Sweep-Secondary Sour.vi"("compliance"=w382, "step"=w385, "error in (no error)"=w391, "total points"=w383, "start"=w384, "VISA session"=w390) -> ("error out"=w389:errorcluster)  [unwired: 1 in]
                          n146 = local write "error?"(w389) -> ()
                        }
                      }
                    }
                    frame True {
                      n147 = local read "Mode"() -> (w403:u16)
                      n148 = call "compliancevi3subvi.vi"("compliance (A)"=w399, "start"=w394, "compliance (V)"=w398, "total points"=w397, "step"=w393, "Mode"=w403) -> ("total points 2"=w396:u16, "compliance"=w395:dbl)  [unwired: 1 in, 1 out]
                      n149 = call "HP415xA _Config-Sweep-Secondary Sour.vi"("compliance"=w395, "step"=w393, "error in (no error)"=w402, "total points"=w396, "start"=w394, "VISA session"=w401) -> ("error out"=w400:errorcluster)  [unwired: 1 in]
                      n150 = local write "error?"(w400) -> ()
                    }
                  }
                }
              }
            }
            frame True {
              w413 = u16 2 items=["disabled", "Var1", "Var2", "Var1'", "Constant"] ("Function")
              n151 = local read "Mode 2"() -> (w422:u16)
              n152 = local read "Function"() -> (w412:u16)
              n153 = call "compliancesubvi2.vi"("compliance (V)"=w420, "Mode"=w422, "compliance (A)"=w421) -> ("compliance"=w423:dbl)  [unwired: 3 in, 1 out]
              n154 = local read "error?"() -> (w414:errorcluster)
              n155 = Equal?(x=w412, y=w413) -> (x = y?=w411:bool)
              n156 = call "HP415xA _Config-Sweep-Primary Sour.vi"("step (linear only)"=w416, "stop"=w415, "start"=w417, "compliance"=w423, "error in (no error)"=w414, "sweep mode"=w419, "sweep spacing (linear: 0)"=w418, "VISA session"=w407) -> ("error out"=w406:errorcluster)  [unwired: 2 in]
              n157 = case shown="False" w411 {
                tunnel: w410 -> [w429 w472]
                tunnel: w409 -> [w428 w471]
                tunnel: w408 -> [w426 w467]
                tunnel: w407 -> [w431 w477]
                tunnel: w406 -> [w425 w476]
                tunnel: w405 -> [w427 w473]
                tunnel: w404 -> [w424 w469]
                frame False {
                  w433 = u16 2 items=["disabled", "Var1", "Var2", "Var1'", "Constant"] ("Function")
                  n158 = local read "Function 3"() -> (w432:u16)
                  n159 = Equal?(x=w432, y=w433) -> (x = y?=w430:bool)
                  n160 = case shown="True" w430 {
                    tunnel: w431 -> [w439 w465]
                    tunnel: w429 -> [w438 w462]
                    tunnel: w428 -> [w436 w460]
                    tunnel: w427 -> [w437 w461]
                    tunnel: w426 -> [w434 w458]
                    tunnel: w425 -> [w440 w464]
                    tunnel: w424 -> [w435 w456]
                    frame False {
                      w443 = u16 2 items=["disabled", "Var1", "Var2", "Var1'", "Constant"] ("Function")
                      n161 = local read "Function 4"() -> (w442:u16)
                      n162 = Equal?(x=w442, y=w443) -> (x = y?=w441:bool)
                      n163 = case shown="True" w441 {
                        tunnel: w440 -> [w444 w455]
                        tunnel: w439 -> [_ w454]
                        tunnel: w438 -> [_ w451]
                        tunnel: w437 -> [_ w452]
                        tunnel: w436 -> [_ w450]
                        tunnel: w435 -> [_ w446]
                        tunnel: w434 -> [_ w447]
                        frame False {
                          n164 = local write "error?"(w444) -> ()
                        }
                        frame True {
                          n165 = local read "Mode 4"() -> (w449:u16)
                          n166 = call "compliancevi3subvi.vi"("compliance (A)"=w451, "start"=w447, "compliance (V)"=w450, "total points"=w452, "step"=w446, "Mode"=w449) -> ("total points 2"=w448:u16, "compliance"=w445:dbl)  [unwired: 1 in, 1 out]
                          n167 = call "HP415xA _Config-Sweep-Secondary Sour.vi"("compliance"=w445, "step"=w446, "error in (no error)"=w455, "total points"=w448, "start"=w447, "VISA session"=w454) -> ("error out"=w453:errorcluster)  [unwired: 1 in]
                          n168 = local write "error?"(w453) -> ()
                        }
                      }
                    }
                    frame True {
                      n169 = local read "Mode 3"() -> (w466:u16)
                      n170 = call "compliancevi3subvi.vi"("compliance (A)"=w462, "start"=w458, "compliance (V)"=w460, "total points"=w461, "step"=w456, "Mode"=w466) -> ("total points 2"=w459:u16, "compliance"=w457:dbl)  [unwired: 1 in, 1 out]
                      n171 = call "HP415xA _Config-Sweep-Secondary Sour.vi"("compliance"=w457, "step"=w456, "error in (no error)"=w464, "total points"=w459, "start"=w458, "VISA session"=w465) -> ("error out"=w463:errorcluster)  [unwired: 1 in]
                      n172 = local write "error?"(w463) -> ()
                    }
                  }
                }
                frame True {
                  n173 = local read "Mode"() -> (w474:u16)
                  n174 = call "compliancevi3subvi.vi"("compliance (A)"=w472, "start"=w467, "compliance (V)"=w471, "total points"=w473, "step"=w469, "Mode"=w474) -> ("total points 2"=w468:u16, "compliance"=w470:dbl)  [unwired: 1 in, 1 out]
                  n175 = call "HP415xA _Config-Sweep-Secondary Sour.vi"("compliance"=w470, "step"=w469, "error in (no error)"=w476, "total points"=w468, "start"=w467, "VISA session"=w477) -> ("error out"=w475:errorcluster)  [unwired: 1 in]
                  n176 = local write "error?"(w475) -> ()
                }
              }
            }
          }
        }
        frame True {
          w486 = u16 2 items=["disabled", "Var1", "Var2", "Var1'", "Constant"] ("Function 2")
          n177 = local read "Mode"() -> (w496:u16)
          n178 = local read "Function 2"() -> (w487:u16)
          n179 = call "compliancesubvi2.vi"("compliance (V)"=w495, "Mode"=w496, "compliance (A)"=w494) -> ("compliance"=w497:dbl)  [unwired: 3 in, 1 out]
          n180 = local read "error?"() -> (w488:errorcluster)
          n181 = Equal?(x=w487, y=w486) -> (x = y?=w485:bool)
          n182 = call "HP415xA _Config-Sweep-Primary Sour.vi"("step (linear only)"=w491, "stop"=w490, "start"=w489, "compliance"=w497, "error in (no error)"=w488, "sweep mode"=w492, "sweep spacing (linear: 0)"=w493, "VISA session"=w478) -> ("error out"=w479:errorcluster)  [unwired: 2 in]
          n183 = case shown="True" w485 {
            tunnel: w484 -> [w503 w547]
            tunnel: w483 -> [w504 w546]
            tunnel: w482 -> [w501 w543]
            tunnel: w481 -> [w502 w545]
            tunnel: w480 -> [w500 w541]
            tunnel: w479 -> [w499 w550]
            tunnel: w478 -> [w498 w548]
            frame False {
              w507 = u16 2 items=["disabled", "Var1", "Var2", "Var1'", "Constant"] ("Function 2")
              n184 = local read "Function 3"() -> (w506:u16)
              n185 = Equal?(x=w506, y=w507) -> (x = y?=w505:bool)
              n186 = case shown="True" w505 {
                tunnel: w504 -> [w512 w530]
                tunnel: w503 -> [w513 w531]
                tunnel: w502 -> [w510 w536]
                tunnel: w501 -> [w511 w533]
                tunnel: w500 -> [w509 w532]
                tunnel: w499 -> [w514 w539]
                tunnel: w498 -> [w508 w537]
                frame False {
                  w517 = u16 2 items=["disabled", "Var1", "Var2", "Var1'", "Constant"] ("Function 2")
                  n187 = local read "Function 4"() -> (w516:u16)
                  n188 = Equal?(x=w516, y=w517) -> (x = y?=w515:bool)
                  n189 = case shown="True" w515 {
                    tunnel: w514 -> [w518 w529]
                    tunnel: w513 -> [_ w519]
                    tunnel: w512 -> [_ w520]
                    tunnel: w511 -> [_ w521]
                    tunnel: w510 -> [_ w526]
                    tunnel: w509 -> [_ w523]
                    tunnel: w508 -> [_ w527]
                    frame False {
                      n190 = local write "error?"(w518) -> ()
                    }
                    frame True {
                      n191 = local read "Mode 4"() -> (w525:u16)
                      n192 = call "compliancevi3subvi.vi"("compliance (A)"=w519, "start"=w521, "compliance (V)"=w520, "total points"=w526, "step"=w523, "Mode"=w525) -> ("total points 2"=w522:u16, "compliance"=w524:dbl)  [unwired: 1 in, 1 out]
                      n193 = call "HP415xA _Config-Sweep-Secondary Sour.vi"("compliance"=w524, "step"=w523, "error in (no error)"=w529, "total points"=w522, "start"=w521, "VISA session"=w527) -> ("error out"=w528:errorcluster)  [unwired: 1 in]
                      n194 = local write "error?"(w528) -> ()
                    }
                  }
                }
                frame True {
                  n195 = local read "Mode 3"() -> (w540:u16)
                  n196 = call "compliancevi3subvi.vi"("compliance (A)"=w531, "start"=w533, "compliance (V)"=w530, "total points"=w536, "step"=w532, "Mode"=w540) -> ("total points 2"=w535:u16, "compliance"=w534:dbl)  [unwired: 1 in, 1 out]
                  n197 = call "HP415xA _Config-Sweep-Secondary Sour.vi"("compliance"=w534, "step"=w532, "error in (no error)"=w539, "total points"=w535, "start"=w533, "VISA session"=w537) -> ("error out"=w538:errorcluster)  [unwired: 1 in]
                  n198 = local write "error?"(w538) -> ()
                }
              }
            }
            frame True {
              n199 = local read "Mode 2"() -> (w551:u16)
              n200 = call "compliancevi3subvi.vi"("compliance (A)"=w547, "start"=w543, "compliance (V)"=w546, "total points"=w545, "step"=w541, "Mode"=w551) -> ("total points 2"=w544:u16, "compliance"=w542:dbl)  [unwired: 1 in, 1 out]
              n201 = call "HP415xA _Config-Sweep-Secondary Sour.vi"("compliance"=w542, "step"=w541, "error in (no error)"=w550, "total points"=w544, "start"=w543, "VISA session"=w548) -> ("error out"=w549:errorcluster)  [unwired: 1 in]
              n202 = local write "error?"(w549) -> ()
            }
          }
        }
      }
      n203 = local read "error?"() -> (w191:errorcluster)
      n204 = call "HP415xA _Config-Meas-Timing.vi"("error in (no error)"=w191, "wait time parameter"="wait time parameter", "integration time"="integration time", "VISA session"=w187) -> ("error out"=w190:errorcluster)  [unwired: 2 in]
      n205 = local write "error?"(w190) -> ()
    }
    frame #2 {
      w592 = u32 1 items=["stop  ", "single  ", "single-append  ", "stress start  ", "continuous  ", "standby on  ", "standby off  ", "zero  "] ("function (stop:0)")
      w596 = u16 2 items=["disabled", "Var1", "Var2", "Var1'", "Constant"] ("Function")
      w600 = u16 1 items=["disabled", "Var1", "Var2", "Var1'", "Constant"] ("Function")
      n206 = local read "Function"() -> (w602:u16)
      n207 = local read "Function"() -> (w595:u16)
      n208 = Equal?(x=w602, y=w600) -> (x = y?=w601:bool)
      n209 = Equal?(x=w595, y=w596) -> (x = y?=w594:bool)
      n210 = case shown="False" w601 {
        tunnel: [w910 w925] -> w553
        tunnel: [w911 w924] -> _
        tunnel: w600 -> [w908 _]
        frame False {
          n211 = local read "Function 2"() -> (w912:u16)
          n212 = Equal?(x=w912, y=w908) -> (x = y?=w909:bool)
          n213 = case shown="False" w909 {
            tunnel: [w913 w923] -> w911
            tunnel: [w914 w922] -> w910
            tunnel: w908 -> [w917 _]
            frame False {
              n214 = local read "Function 3"() -> (w916:u16)
              n215 = Equal?(x=w916, y=w917) -> (x = y?=w915:bool)
              n216 = case shown="True" w915 {
                tunnel: [w919 w921] -> w914
                tunnel: [w918 w920] -> w913
                frame False {
                  n217 = local read "Vname 4"() -> (w919:string)
                  n218 = local read "Iname 4"() -> (w918:string)
                }
                frame True {
                  n219 = local read "Vname 3"() -> (w921:string)
                  n220 = local read "Iname 3"() -> (w920:string)
                }
              }
            }
            frame True {
              n221 = local read "Iname 2"() -> (w923:string)
              n222 = local read "Vname 2"() -> (w922:string)
            }
          }
        }
        frame True {
          n223 = local read "Vname"() -> (w925:string)
          n224 = local read "Iname"() -> (w924:string)
        }
      }
      n225 = case shown="False" w594 {
        tunnel: [w852 w905] -> w559
        tunnel: [w851 TRUE ("x = y?")] -> w555
        frame False {
          w855 = u16 2 items=["disabled", "Var1", "Var2", "Var1'", "Constant"] ("Function")
          n226 = local read "Function 2"() -> (w854:u16)
          n227 = Equal?(x=w854, y=w855) -> (x = y?=w853:bool)
          n228 = case shown="False" w853 {
            tunnel: [w857 w895] -> w852
            tunnel: [w856 TRUE ("x = y?")] -> w851
            frame False {
              w860 = u16 2 items=["disabled", "Var1", "Var2", "Var1'", "Constant"] ("Function")
              n229 = local read "Function 3"() -> (w859:u16)
              n230 = Equal?(x=w859, y=w860) -> (x = y?=w858:bool)
              n231 = case shown="False" w858 {
                tunnel: [w865 w885] -> w857
                tunnel: [w861 TRUE ("x = y?")] -> w856
                frame False {
                  w864 = u16 2 items=["disabled", "Var1", "Var2", "Var1'", "Constant"] ("Function")
                  n232 = local read "Function 4"() -> (w863:u16)
                  n233 = Equal?(x=w863, y=w864) -> (x = y?=w862:bool)
                  n234 = case shown="True" w862 {
                    tunnel: ["0" ("Vname 4") w875] -> w865
                    tunnel: [FALSE ("x = y?") TRUE ("x = y?")] -> w861
                    frame False {
                    }
                    frame True {
                      w869 = u16 2 items=["V", "I", "VPulse", "IPulse", "Common"] ("Mode 2")
                      w872 = u16 0 items=["V", "I", "VPulse", "IPulse", "Common"] ("Mode 2")
                      n235 = local read "Mode 4"() -> (w871:u16)
                      n236 = Equal?(x=w872, y=w871) -> (x = y?=w873:bool)
                      n237 = Equal?(x=w871, y=w869) -> (x = y?=w870:bool)
                      n238 = Or(x=w873, y=w870) -> (x .or. y?=w868:bool)
                      n239 = case shown="True" w868 {
                        tunnel: [w876 w877] -> w875
                        frame False {
                          n240 = local read "Iname 4"() -> (w876:string)
                        }
                        frame True {
                          n241 = local read "Vname 4"() -> (w877:string)
                        }
                      }
                    }
                  }
                }
                frame True {
                  w881 = u16 2 items=["V", "I", "VPulse", "IPulse", "Common"] ("Mode 2")
                  w880 = u16 0 items=["V", "I", "VPulse", "IPulse", "Common"] ("Mode 2")
                  n242 = local read "Mode 3"() -> (w879:u16)
                  n243 = Equal?(x=w880, y=w879) -> (x = y?=w883:bool)
                  n244 = Equal?(x=w879, y=w881) -> (x = y?=w882:bool)
                  n245 = Or(x=w883, y=w882) -> (x .or. y?=w878:bool)
                  n246 = case shown="False" w878 {
                    tunnel: [w886 w887] -> w885
                    frame False {
                      n247 = local read "Iname 3"() -> (w886:string)
                    }
                    frame True {
                      n248 = local read "Vname 3"() -> (w887:string)
                    }
                  }
                }
              }
            }
            frame True {
              w889 = u16 2 items=["V", "I", "VPulse", "IPulse", "Common"] ("Mode 2")
              w890 = u16 0 items=["V", "I", "VPulse", "IPulse", "Common"] ("Mode 2")
              n249 = local read "Mode 2"() -> (w891:u16)
              n250 = Equal?(x=w890, y=w891) -> (x = y?=w893:bool)
              n251 = Equal?(x=w891, y=w889) -> (x = y?=w892:bool)
              n252 = Or(x=w893, y=w892) -> (x .or. y?=w888:bool)
              n253 = case shown="True" w888 {
                tunnel: [w896 w897] -> w895
                frame False {
                  n254 = local read "Iname 2"() -> (w896:string)
                }
                frame True {
                  n255 = local read "Vname 2"() -> (w897:string)
                }
              }
            }
          }
        }
        frame True {
          w902 = u16 2 items=["V", "I", "VPulse", "IPulse", "Common"] ("Mode")
          w903 = u16 0 items=["V", "I", "VPulse", "IPulse", "Common"] ("Mode")
          n256 = local read "Mode"() -> (w901:u16)
          n257 = Equal?(x=w901, y=w903) -> (x = y?=w900:bool)
          n258 = Equal?(x=w901, y=w902) -> (x = y?=w899:bool)
          n259 = Or(x=w900, y=w899) -> (x .or. y?=w898:bool)
          n260 = case shown="True" w898 {
            tunnel: [w906 w907] -> w905
            frame False {
              n261 = local read "Iname"() -> (w906:string)
            }
            frame True {
              n262 = local read "Vname"() -> (w907:string)
            }
          }
        }
      }
      n263 = local read "error?"() -> (w584:errorcluster)
      n264 = Unbundle("Y2 axis settings") -> ("Y2 axis on/off"=w578:bool, "MINIMUM"=w589:ext, "MAXIMUM"=w588:ext, "Variable name"=w554:string, "LIN or LOG axis"=w587:string)
      n265 = local read "Var2 step settings"() -> (w598:T6)
      n266 = local read "Var1 sweep settings"() -> (w599:T7)
      n267 = local read "VISA session"() -> (w571:refnum<visa-resource-name>)
      n268 = call "Y1subvi.vi"("MAXIMUM"="MAXIMUM", "Variable name"="Y1 axis", "error in (no error)"=w584, "MINIMUM"="MINIMUM", "LIN or LOG axis"="LIN", "VISA resource name"=w571) -> ("error out"=w585:errorcluster)
      n269 = case shown="False" w578 {
        tunnel: w585 -> [w843 w850]
        tunnel: w571 -> [_ w849]
        tunnel: w589 -> [_ w848]
        tunnel: w588 -> [_ w847]
        tunnel: w554 -> [_ w846]
        tunnel: w587 -> [_ w845]
        tunnel: [w843 w844] -> w586
        frame False {
        }
        frame True {
          n270 = call "Y2subvi.vi"("MAXIMUM"=w847, "Variable name"=w846, "error in (no error)"=w850, "MINIMUM"=w848, "LIN or LOG axis"=w845, "VISA resource name"=w849) -> ("error out"=w844:errorcluster)
        }
      }
      n271 = Unbundle(w598) -> ("total points"=w597:u16)  [unwired: 4 out]
      n272 = Decrement(x=w597) -> (x-1=w562:u16)
      n273 = Unbundle(w599) -> ("start"=w570:dbl)  [unwired: 6 out]
      n274 = call "HP415xA Op-Start-Stop.vi"("error in (no error)"=w586, "function (stop:0)"=w592, "wait until finish"=TRUE, "VISA session"=w571) -> ("error out"=w591:errorcluster)  [unwired: 6 in, 1 out]
      n275 = call "HP415xA Op-Download Trace.vi"("error in (no error)"=w591, "trace (variable) name"=w553, "VISA session"=w571) -> ("error out"=w605:errorcluster, "trace"=w576:dbl[])
      n276 = call "HP415xA Op-Download Trace.vi"("error in (no error)"=w605, "trace (variable) name"="Y1 axis", "VISA session"=w571) -> ("error out"=w581:errorcluster, "trace"=w572:dbl[])
      n277 = case shown="True" w578 {
        tunnel: w581 -> [w827 w836]
        tunnel: w571 -> [_ w835]
        tunnel: w554 -> [_ w834]
        tunnel: [w827 w833] -> w573
        tunnel: w576 -> [w825 w832]
        tunnel: w572 -> [w826 w831]
        tunnel: [w824 w830] -> w558
        tunnel: [dbl[] [] ("trace") w829] -> w577
        tunnel: [cluster{"trace":dbl[], "trace":dbl[]} {"trace"=[], "trace"=[]} w828] -> w556
        frame False {
          n278 = Bundle("trace"=w825, "trace"=w826) -> (w824:cluster{"trace":dbl[], "trace":dbl[]})  [unwired: 1 in]
        }
        frame True {
          n279 = call "HP415xA Op-Download Trace.vi"("error in (no error)"=w836, "trace (variable) name"=w834, "VISA session"=w835) -> ("error out"=w833:errorcluster, "trace"=w829:dbl[])
          n280 = stacked-sequence {
            tunnel: w829 -> [_ w842]
            tunnel: w832 -> [w839 w841]
            tunnel: w831 -> [w838 _]
            tunnel: [w837 _] -> w830
            tunnel: [_ w840] -> w828
            frame #0 {
              n281 = Bundle("trace"=w839, "trace"=w838) -> (w837:cluster{"trace":dbl[], "trace":dbl[]})  [unwired: 1 in]
            }
            frame #1 {
              n282 = Bundle("trace"=w841, "trace"=w842) -> (w840:cluster{"trace":dbl[], "trace":dbl[]})  [unwired: 1 in]
              "Gate Current Plot" <- w840
            }
          }
        }
      }
      "graphic display" <- w558
      n283 = Build Array(w556) -> (w557:cluster{"trace":dbl[], "trace":dbl[]}[])
      n284 = case shown="True" w555 {
        tunnel: w570 -> [_ w732]
        tunnel: w572 -> [w610 w731]
        tunnel: w576 -> [w611 w730]
        tunnel: w562 -> [_ w729]
        tunnel: w571 -> [_ w725]
        tunnel: w573 -> [_ w724]
        tunnel: [w612 w616] -> w575
        tunnel: w559 -> [_ w723]
        tunnel: w559 -> [_ w718]
        tunnel: [dbl[] [] ("trace") w722] -> w574
        tunnel: w569 -> [_ w626]
        tunnel: w568 -> [_ w624]
        tunnel: w567 -> [_ w623]
        tunnel: [_ w635] -> w566
        tunnel: [_ w630] -> w565
        tunnel: w564 -> [_ w701]
        tunnel: w563 -> [_ w700]
        tunnel: w562 -> [_ _]
        tunnel: w561 -> [_ _]
        tunnel: w560 -> [_ w684]
        tunnel: w557 -> [_ w627]
        tunnel: [_ w619] -> w552
        frame False {
          n285 = Build Array(w611, w610) -> (w607:dbl[][])
          n286 = local read "error? 2"() -> (w612:errorcluster)
          n287 = call-poly <vilib>:"Write To Spreadsheet File.vi"("transpose? (no:F)"=TRUE ("append to file? (new file:F)"), "format (%.3f)"="%.5e", "2D data"=w607) -> ()  [unwired: 5 in, 1 out]
        }
        frame True {
          (unwired) "\r"
          w622 = "\r"
          w625 = "\r"
          # "Find Smallest Vd Value"
          # "Picks linear Id based on Smallest Vd"
          # "Dielectric"
          # "Data Values"
          # "Headers"
          n288 = call "HP415xA Op-Download Trace.vi"("error in (no error)"=w724, "trace (variable) name"=w723, "VISA session"=w725) -> ("error out"=w616:errorcluster, "trace"=w722:dbl[])
          n289 = Initialize Array("") -> (w702:string[])  [unwired: 1 in]
          n290 = for {
            N: w729 -> [w733]
            shift-right: [w750] -> w635
            shift-left: w730 -> [w746]
            tunnel: w732 -> [w752]
            tunnel: [w751] -> _ mode=indexing
            shift-right: [w747] -> w630
            shift-left: w731 -> [w749]
            tunnel: [w748] -> w678 mode=indexing
            shift-right: [w743] -> w621
            shift-left: w722 -> [w745]
            tunnel: w718 -> [_]
            tunnel: [w737] -> w679 mode=indexing
            shift-right: [w736] -> w706
            shift-left: w702 -> [w735]
            tunnel: [w733] -> _ mode=indexing
            # "Cuts data at each new loop"
            # "Id Data"
            # "Vd Data"
            # "Vg Data"
            n291 = Search 1D Array(1D array=w746, element=w752, start index (0)=1) -> (index of element=w744:i32)
            n292 = Split 1D Array(array=w745, index=w744) -> (first subarray=w741:dbl[], second subarray=w743:dbl[])
            n293 = Split 1D Array(array=w746, index=w744) -> (first subarray=w751:dbl[], second subarray=w750:dbl[])
            n294 = Split 1D Array(array=w749, index=w744) -> (first subarray=w748:dbl[], second subarray=w747:dbl[])
            n295 = Array Size(array=w741) -> (size(s)=w740:i32)
            n296 = Decrement(x=w740) -> (x-1=w739:i32)
            n297 = Array Subset(array=w741, index=w739) -> (w742:dbl[])  [unwired: 1 in]
            n298 = Number To Exponential String(number=w742) -> (E-format string=w738:string[])  [unwired: 3 in]
            n299 = Build Array (concatenate)("Id", w735) -> (w736:string[])
            n300 = Concatenate Strings(w738) -> (w737:string)
          }
          n301 = call "TempHumSample.vi"("VISA resource name"=refnum<visa-resource-name> "COM4", "error in (no error)"=w616) -> ("CurHum"=w614:dbl, "CurTemp"=w613:dbl)  [unwired: 6 in, 1 out]
          n302 = Fract/Exp String To Number(string=w700) -> (number=w682:dbl)  [unwired: 3 in, 1 out]
          n303 = Fract/Exp String To Number(string=w701) -> (number=w683:dbl)  [unwired: 3 in, 1 out]
          n304 = local read "Temp (K)"() -> (w674:dbl)
          n305 = local read "NumPts"() -> (w681:dbl)
          n306 = local read "NumPts"() -> (w675:dbl)
          n307 = Fract/Exp String To Number(string=w684) -> (number=w676:dbl)  [unwired: 3 in, 1 out]
          n308 = Array Size(array=w621) -> (size(s)=w716:i32)
          n309 = call "STS Calculator.vi"("NumPts"=w675, "Saturation Id"=w630, "Vg Column"=w635) -> ("Sub Threshold Swing"=w668:dbl)  [unwired: 5 in, 3 out]
          n310 = call "Mobility-Vt Calculator_Saturation_12_09_10a_JW.vi"("Vg Column"=w635, "Dielectric Constant"="Dielectric Constant", "Sat Id Column"=w630, "NumPts"=w675, "Length"=w682, "Width"=w683, "Dielectric Thickness"=w676) -> ("Check Cluster"=w664:T8, "Mobility-Sat"=w673:dbl, "VT-Sat"=w669:dbl, "Off I-Sat"=w670:dbl, "On/Off I-Sat"=w671:dbl)  [unwired: 4 out]
          n311 = local write "Check Cluster"(w664) -> ()
          n312 = Decrement(x=w716) -> (x-1=w715:i32)
          n313 = call "Trap Density_VT.vi"("VT"=w669, "Dielectric"=w676) -> ("Trap Density-VT"=w667:dbl)
          n314 = call "Trap Density_STS.vi"("Temp (T) [K]"=w674, "S.T.S. (S)"=w668, "Dielectric"=w676) -> ("Trap Density (N)"=w666:dbl)  [unwired: 8 in]
          n315 = Array Subset(array=w621, index=w715) -> (w714:dbl[])  [unwired: 1 in]
          n316 = Number To Exponential String(number=w714) -> (E-format string=w710:string[])  [unwired: 3 in]
          n317 = Build Array("Sample Temp (K):", "RH (%):", "", "Mobility-Sat (cm^2/Vs):", "Mobility-Lin (cm^2/Vs):", "On/Off I-Sat:", "Off I-Sat (A):", "Vt-Sat (V):", "STS-Sat (V/decade):", "Trap Density-VT (Traps/Vcm^2):", "Trap Density-STS (Traps/Vcm^2):") -> (w698:string[])
          n318 = Build Array (concatenate)(w635, w678, w630) -> (w728:dbl[][])
          n319 = Concatenate Strings(w710) -> (w620:string)
          n320 = Build Array (concatenate)(w679, w620) -> (w677:string[])
          n321 = Fract/Exp String To Number(string=w677) -> (number=w662:dbl[])  [unwired: 3 in, 1 out]
          n322 = Build Array (concatenate)(w678, w630) -> (w660:dbl[][])
          n323 = Build Array("Vg", "Id") -> (w707:string[])
          n324 = Absolute Value(x=w662) -> (abs(x)=w663:dbl[])
          n325 = Insert Into Array(array=w707, index=2, new element=w706) -> (w705:string[])
          n326 = Array Max & Min(array=w663) -> (min index (indices)=w659:i32)  [unwired: 3 out]
          n327 = Index Array(array=w662, index=w659) -> (element=w661:dbl)
          n328 = Transpose 2D Array(2D array=w728) -> (transposed array=w726:dbl[][])
          n329 = Build Array (concatenate)("Vd=", w679, w620) -> (w713:string[])
          n330 = Index Array(array=w660, index (row)=w659) -> (element=w632:dbl[])  [unwired: 1 in]
          n331 = call "Mobility-Vt Calculator_Linear.vi"("Vg Column"=w635, "Vd"=w661, "Lin Id Column"=w632, "NumPts"=w681, "Length"=w682, "Width"=w683, "Dielectric Thickness"=w676, "Dielectric Constant"="Dielectric Constant") -> ("Mobility-Lin"=w672:dbl)  [unwired: 1 in, 6 out]
          n332 = Build Array(w613, w614, w673, w672, w671, w670, w669, w668, w667, w666) -> (w697:dbl[])
          n333 = Number To Exponential String(number=w697) -> (E-format string=w657:string[])  [unwired: 3 in]
          n334 = Bundle("Mobility-Sat"=w673, "Mobility-Lin"=w672, "On/Off I-Sat"=w671, "Off I-Sat"=w670, "VT-Sat"=w669, "Sub Threshold Swing"=w668, "Trap Density-VT"=w667, "Trap Density (N)"=w666) -> (w665:T9)  [unwired: 1 in]
          n335 = local write "Output"(w665) -> ()
          n336 = Insert Into Array(array=w657, index=1, new element="") -> (w654:string[])
          n337 = Build Array(w698, w654) -> (w653:string[][])
          n338 = Transpose 2D Array(2D array=w653) -> (transposed array=w652:string[][])
          n339 = Array To Spreadsheet String(array=w713, 3:"%s") -> (spreadsheet string=w717:string)  [unwired: 1 in]
          n340 = Array To Spreadsheet String(array=w705, 3:"%s") -> (spreadsheet string=w711:string)  [unwired: 1 in]
          n341 = Array To Spreadsheet String(array=w652, 3:"%s") -> (spreadsheet string=w695:string)  [unwired: 1 in]
          n342 = Array To Spreadsheet String(array=w726, 3:"%.5e" ("format string")) -> (spreadsheet string=w719:string)  [unwired: 1 in]
          n343 = Concatenate Strings(w626, w625, w624, w625, w623, w695, w625, w717, w711, w719, w622) -> (w721:string)
          n344 = Absolute Value(x=w632) -> (abs(x)=w637:dbl[])
          n345 = Absolute Value(x=w630) -> (abs(x)=w634:dbl[])
          n346 = Absolute Value(x=w632) -> (abs(x)=w631:dbl[])
          n347 = Absolute Value(x=w630) -> (abs(x)=w629:dbl[])
          n348 = Square Root(x=w637) -> (sqrt(x)=w636:dbl[])
          n349 = Square Root(x=w634) -> (sqrt(x)=w633:dbl[])
          n350 = Concatenate Strings(w626, w625, w624, w622, w623, w622) -> (w619:string)
          n351 = local read "Input Path"() -> (w685:path)
          n352 = Bundle("trace"=w635, w631) -> (w640:cluster{"trace":dbl[], dbl[]})  [unwired: 1 in]
          n353 = Bundle("trace"=w635, w629) -> (w643:cluster{"trace":dbl[], dbl[]})  [unwired: 1 in]
          n354 = Bundle("trace"=w635, w636) -> (w639:cluster{"trace":dbl[], dbl[]})  [unwired: 1 in]
          n355 = Bundle("trace"=w635, w633) -> (w644:cluster{"trace":dbl[], dbl[]})  [unwired: 1 in]
          n356 = Bundle("trace"=w635, w632) -> (w646:cluster{"trace":dbl[], dbl[]})  [unwired: 1 in]
          n357 = Bundle("trace"=w635, "trace"=w630) -> (w648:cluster{"trace":dbl[], "trace":dbl[]})  [unwired: 1 in]
          n358 = Build Array(w639) -> (w638:cluster{"trace":dbl[], dbl[]}[])
          n359 = Build Array(w640) -> (w628:cluster{"trace":dbl[], dbl[]}[])
          n360 = Build Array(w644) -> (w641:cluster{"trace":dbl[], dbl[]}[])
          n361 = Build Array(w643) -> (w642:cluster{"trace":dbl[], dbl[]}[])
          n362 = Build Array(w646) -> (w645:cluster{"trace":dbl[], dbl[]}[])
          n363 = Build Array(w648) -> (w647:cluster{"trace":dbl[], "trace":dbl[]}[])
          n364 = local read "Graph Cluster"() -> (w650:T1)
          n365 = Bundle By Name(cluster=w650, "Linear Sqrt"=w638, "Linear Log"=w628, "Linear Raw"=w645, "Saturation Sqrt"=w641, "Saturation Log"=w642, "Saturation Raw"=w647, "Gate Current"=w627) -> (w649:T1)
          n366 = call <vilib>:"Write Characters To File.vi"("append to file? (new file:F)"=TRUE, "character string"=w721, "file path (dialog if empty)"=w685) -> ("new file path (Not A Path if cancelled)"=w693:path)  [unwired: 2 in]
          n367 = local write "Output Path"(w693) -> ()
          n368 = local write "Graph Cluster"(w649) -> ()
        }
      }
      n369 = case shown="True" w578 {
        tunnel: w562 -> [_ w762]
        tunnel: w555 -> [_ w763]
        tunnel: w576 -> [_ w761]
        tunnel: w570 -> [_ w760]
        tunnel: w577 -> [_ w759]
        tunnel: w574 -> [_ w758]
        tunnel: w559 -> [_ w757]
        tunnel: w554 -> [_ w756]
        tunnel: w553 -> [_ w755]
        tunnel: w552 -> [_ w754]
        frame False {
        }
        frame True {
          n370 = case shown="True" w763 {
            tunnel: w762 -> [_ w792]
            tunnel: w761 -> [w767 w804]
            tunnel: w760 -> [_ w803]
            tunnel: w759 -> [w768 w802]
            tunnel: w758 -> [_ w801]
            tunnel: w757 -> [_ w789]
            tunnel: w756 -> [_ w782]
            tunnel: w755 -> [_ w781]
            tunnel: w754 -> [_ w770]
            frame False {
              n371 = Build Array(w767, w768) -> (w766:dbl[][])
              n372 = call-poly <vilib>:"Write To Spreadsheet File.vi"("transpose? (no:F)"=TRUE, "format (%.3f)"="%.5e", "2D data"=w766) -> ()  [unwired: 5 in, 1 out]
            }
            frame True {
              n373 = for {
                N: w792 -> [_]
                shift-right: [w818] -> w800
                shift-left: w804 -> [w819]
                tunnel: w803 -> [w821]
                tunnel: [w817] -> _ mode=indexing
                shift-right: [w814] -> w784
                shift-left: w802 -> [w816]
                tunnel: [w815] -> w799 mode=indexing
                shift-right: [w811] -> w796
                shift-left: w801 -> [w812]
                tunnel: [w808] -> w793 mode=indexing
                shift-right: [w807] -> w783
                shift-left: _ -> [w806]
                tunnel: w782 -> [w805]
                n374 = Search 1D Array(1D array=w819, element=w821, start index (0)=1) -> (index of element=w813:i32)
                n375 = Split 1D Array(array=w819, index=w813) -> (first subarray=w817:dbl[], second subarray=w818:dbl[])
                n376 = Split 1D Array(array=w816, index=w813) -> (first subarray=w815:dbl[], second subarray=w814:dbl[])
                n377 = Split 1D Array(array=w812, index=w813) -> (first subarray=w809:dbl[], second subarray=w811:dbl[])
                n378 = Index Array(array=w809, index=1) -> (element=w808:dbl)
                n379 = Build Array (concatenate)(w805, w806) -> (w807:string[])
              }
              n380 = Build Array (concatenate)(w800, w799, w784) -> (w798:dbl[][])
              n381 = Index Array(array=w796, index=1) -> (element=w794:dbl)
              n382 = Transpose 2D Array(2D array=w798) -> (transposed array=w797:dbl[][])
              n383 = Insert Into Array(array=w793, index=w792, new element=w794) -> (w791:dbl[])
              n384 = Array To Spreadsheet String(array=w791, 3:"%.5e" ("format string")) -> (spreadsheet string=w778:string)  [unwired: 1 in]
              n385 = Concatenate Strings(w789, "= " ("string")) -> (w779:string)
              n386 = Array To Spreadsheet String(array=w797, 3:"%.5e" ("format string")) -> (spreadsheet string=w776:string)  [unwired: 1 in]
              n387 = Build Array(w781, w782) -> (w786:string[])
              n388 = Insert Into Array(array=w786, index=2, new element=w783) -> (w785:string[])
              n389 = Concatenate Strings(w779, w778) -> (w777:string)
              n390 = Array To Spreadsheet String(array=w785, 3:"%s") -> (spreadsheet string=w775:string)  [unwired: 1 in]
              n391 = Concatenate Strings(w777, w775, w776) -> (w769:string)
              "concatenated string" <- w769
              n392 = Concatenate Strings(w770, w769) -> (w772:string)
              n393 = local read "LKG Path"() -> (w771:path)
              n394 = call <vilib>:"Write Characters To File.vi"("append to file? (new file:F)"=TRUE, "character string"=w772, "file path (dialog if empty)"=w771) -> ()  [unwired: 2 in, 1 out]
            }
          }
        }
      }
      n395 = call "HP415xA Sys-Error Query.vi"("VISA session"=w571, "error in (no error)"=w575) -> ("error out"=w603:errorcluster)  [unwired: 2 in, 1 out]
      n396 = call "HP415xA  Close.vi"("error in (no error)"=w603, "VISA session"=w571) -> ("error out"=w604:errorcluster)
      n397 = local write "error?"(w604) -> ()
    }
  }
